vi "TapeDriveControllerCK_MasterSlave (3).vi"() -> ()   [LabVIEW 2011]
uses:
  <vilib>/Utility/error.llb/DialogType.ctl
  <instrlib>/Newport ESP301/Newport ESP301.lvlib
panel:
  out "level(ms)":dbl format="%.4g"
  in  "Tab Control":T1(tab)
  in  "Power Status":bool
  in  "Power Status 2":bool
  in  "Filename":string
  out "Slave Axis":i32
  out "Master Axis":i32
  in  "Release Slaving":bool
  in  "Switch Master Slave":bool
  in  "Interval":i32=1 min=1 max=1000
  in  "Reduction Ratio (0)":dbl min=-1000000.0 max=1000000.0 format="%.6g"
  in  "Turn OFF Slave":bool
  in  "Release Slaving\n after Discon":bool
  in  "VISA resource name":refnum<visa-resource-name>="COM1"
  in  "Connect":bool
  in  "Serial Link (RS232)":enum16{"RS232", "USB"}(ring)
  out "Connected?":bool
  in  "Save sinlge\nPicture":bool
  in  "Save all Shots":bool
  in  "Tab Control 2":T2(tab)=enum."Stepped Group"
  in  "Make Pictures":bool
  in  "Number of Steps":i32=5
  in  "Go steps":bool
  in  "Steplength(ms/mm)":dbl=10.0
  in  "Waittime":u32=800
  out "act. Step":u32=4
  in  "Wait befor picture(ms)":u32=50
  in  "Wait after picture(ms) 2":u32=100
  in  "Step Acc":dbl format="%.6f"
  in  "Step Velo":dbl min=-1000000.0 max=1000000.0 format="%.6g"
  in  "Go steps 2":bool
  in  "Waittime 2":u32
  in  "Wait after\n picture(ms) 2":u32
  out "act. Step 2":u32
  in  "Wait befor\n picture(ms) 2":u32
  in  "Steplength(ms) 2":u32
  in  "Number of Steps 2":i32
  in  "Make Pictures 2":bool
  in  "Stiff Velo":dbl min=-1000000.0 max=1000000.0 format="%.6g"
  in  "Stiff Acc":dbl format="%.6f"
  in  "Go steps 3":bool
  in  "1st Holdmove":dbl=20000.0
  in  "Steplength(ms) 3":dbl=10.0
  in  "Waittime 3":u32=1000
  in  "Wait befor\n picture(ms) 3":u32
  in  "Wait after\n picture(ms) 3":u32
  in  "Make Pictures 3":bool
  out "act. Step 3":u32
  in  "Number of Steps 3":i32=6
  in  "Motionphase":T3(array[cluster])=[{"Group Velocity (units/s)"=500.0, "Group Acceleration\n (0 units/s²) "=2000.0, "Group Vector Jerk\n (0 units/s^3)"=1000.0, "Group Decceleration \n(0 units/s²)"=4000.0, "Position (0 units)"=[50.0, 0.0], "groupInit Delay"=30}, {"Group Velocity (units/s)"=1000.0, "Group Acceleration\n (0 units/s²) "=2000.0, "Group Vector Jerk\n (0 units/s^3)"=4000.0, "Group Decceleration \n(0 units/s²)"=2000.0, "Position (0 units)"=[1000.0, 1000.0], "groupInit Delay"=10}]
  in  "StepMode":enum16{"Use Timing", "Use Encoder"}(ring)
  in  "E Stop":bool
  in  "AXIS":i32(ring)=1 items=["Axis1"=1, "Axis3"=3]
  out "Array":T4(array[cluster])
  in  "Acceleration (0 units/s²)":dbl min=0.0 format="%.4g"
  in  "Max Acceleration (0 units/s²)":dbl min=0.0 max=2000000000.0 format="%.6g"
  in  "Maximum Velocity (0 units/s)":dbl min=0.0 max=2000000000.0 format="%.6g"
  in  "Deceleration (0 units/s²)":dbl min=0.0 format="%.6g"
  in  "Velocity feed-forward gain factor (0)":dbl min=0.0 max=2000000000.0 format="%.6g"
  in  "Velocity (units/s)":dbl min=0.0 format="%.4g"
  in  "Acceleration feed-forward gain factor (0)":dbl min=0.0 max=2000000000.0 format="%.6g"
  in  "DAC Offset (0)":dbl min=-10.0 max=10.0 format="%.6g"
  out "DAC Offsets":dbl[](array[numeric]) format="%_6g"
  in  "Group Acceleration\n (0 units/s²)":dbl=4000.0 min=0.0 format="%.6g"
  in  "Group Velocity (units/s)":dbl=1000.0 min=0.0 format="%.4g"
  in  "Group Vector Jerk\n (0 units/s^3)":dbl=1000.0 min=0.0 max=2000000000.0 format="%.4g"
  in  "Group Decceleration \n(0 units/s²)":dbl=4000.0 min=0.0 format="%.6g"
  in  "Feedback Filter Settings":T5
  out "FilterSetup":T6(array[cluster])
  in  "Cluster":cluster{"Master Axis":i32, "Slave Axis":i32}={"Master Axis"=1, "Slave Axis"=3}
  in  "Encoder\nAxis":i32=2
  out "Remaining States":string
  in  "Get Relation of Slave":bool
  out "Slaves Master":i32
  out "Current State":string
  out "Reduction Ratio":dbl format="%.6g"
  out "Interval (ms)":i32
  in  "Motionphase 2":T3(array[cluster])
  in  "Group Move Comp":bool
  in  "Set Zero":bool
  out "Position (units)":dbl format="%.6g"
  in  "groupInit Delay":u32=50
  in  "Wait before read (0ms)":u32=100
  in  "Send Command":bool
  out "Answer":string
  in  "Command":string
  in  "End Program":bool
  in  "Group Mode":bool
  in  "MOVE MASTER":bool
  out "In Motion?":bool
  in  "MaxMotion":dbl=200000.0
  # "Debug Indicators"
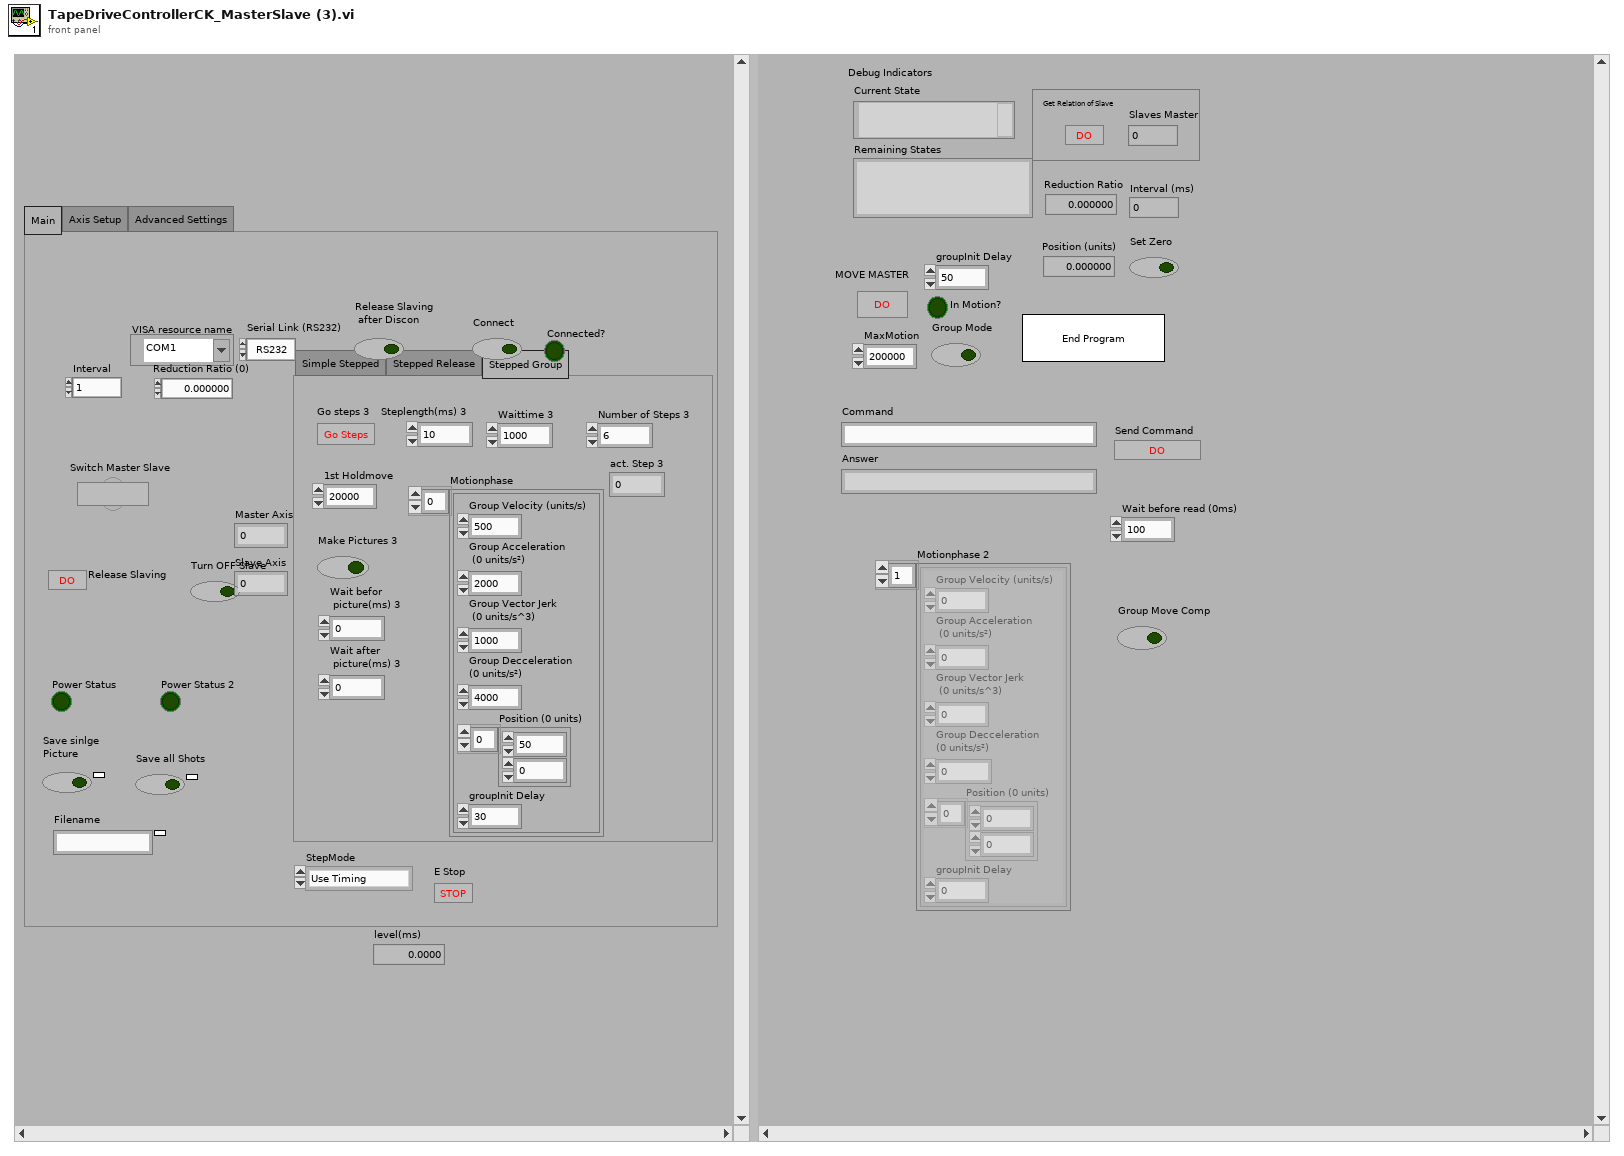
[diagram p1: front panel]
types:
  T1 = enum32{"Main", "Axis Setup", "Advanced Settings"}
  T2 = enum32{"Simple Stepped", "Stepped Release", "Stepped Group"}
  T3 = cluster{"Group Velocity (units/s)":dbl, "Group Acceleration\n (0 units/s²) ":dbl, "Group Vector Jerk\n (0 units/s^3)":dbl, "Group Decceleration \n(0 units/s²)":dbl, "Position (0 units)":dbl[], "groupInit Delay":u32}[]
  T4 = cluster{cluster{"Max Acceleration (units/s²)":dbl, "Maximum Velocity (units/s)":dbl, "Acceleration (units/s²)":dbl, "Deceleration (units/s²)":dbl, "Velocity (units/s)":dbl}, cluster{"Accel Gain":dbl, "Velocity Gain":dbl}}[]
  T5 = cluster{"Ks (0)":dbl, "Ki (0)":dbl, "Kp (0)":dbl, "Kd (0)":dbl}
  T6 = cluster{"Ks":dbl, "Kp":dbl, "Ki":dbl, "Kd":dbl}[]
  T7 = enum32{"invalid app kind", "Development System", "Run Time System", "Student Edition", "Embedded LabVIEW", "Evaluation", "Custom"}
  T8 = enum32{"Invalid", "Standard", "Closed", "Hidden", "Minimized", "Maximized"}
  T9 = enum16{"Trapezoidal Mode", "S-curve Mode", "Jog Mode", "Slave to master's desired position (trajectory)", "Slave to master's actual position (feedback)", "Slave to master's actual velocity for jogging"}
  T10 = cluster{"Grouped?":bool, "Master Axis":i32, "Group Number (1)":i32}
  T11 = cluster{"Core":cluster{"Current VI Reference":refnum<vi>, "Close Panel on Exit?":bool}, "VISA resource name":refnum<visa-resource-name>, "Velocity (units/s)":dbl, "Acceleration (0 units/s²)":dbl, "Connected?":bool, "Master Axis":i32, "Slave Axis":i32, "In Motion?":bool, "Stepper Cluster":cluster{"Stepped Motion":bool, "Moving":bool, "millisecond timer value":u32, "act. Step":u32}, "Stepper Cluster 2":cluster{"Stepped Motion":bool, "Moving":bool, "millisecond timer value":u32, "act. Step":u32}, "Group Cluster":cluster{"Grouped?":bool, "Master Axis":i32, "Group Number (1)":i32}, "Stepper Cluster 3":cluster{"Stepped Motion":bool, "Moving":bool, "millisecond timer value":u32, "act. Step":u32}, "Stepper Cluster 4":cluster{"Stepped Motion":bool, "Moving":bool, "millisecond timer value":u32, "act. Step":u32}, "actual Position":dbl, "Last Position":dbl}
  T12 = typedef "DialogType.ctl" = u16
  T13 = cluster{"Stepped Motion":bool, "Moving":bool, "millisecond timer value":u32, "act. Step":u32}
  T14 = cluster{"Current VI Reference":refnum<vi>, "Close Panel on Exit?":bool}
  T15 = cluster{"Acceleration (units/s²)":dbl, "Maximum Velocity (units/s)":dbl, "Acceleration (units/s²)":dbl, "Deceleration (units/s²)":dbl, "Velocity (units/s)":dbl}
  T16 = cluster{cluster{"Acceleration (units/s²)":dbl, "Maximum Velocity (units/s)":dbl, "Acceleration (units/s²)":dbl, "Deceleration (units/s²)":dbl, "Velocity (units/s)":dbl}, cluster{"Gain":dbl, "Gain":dbl}}
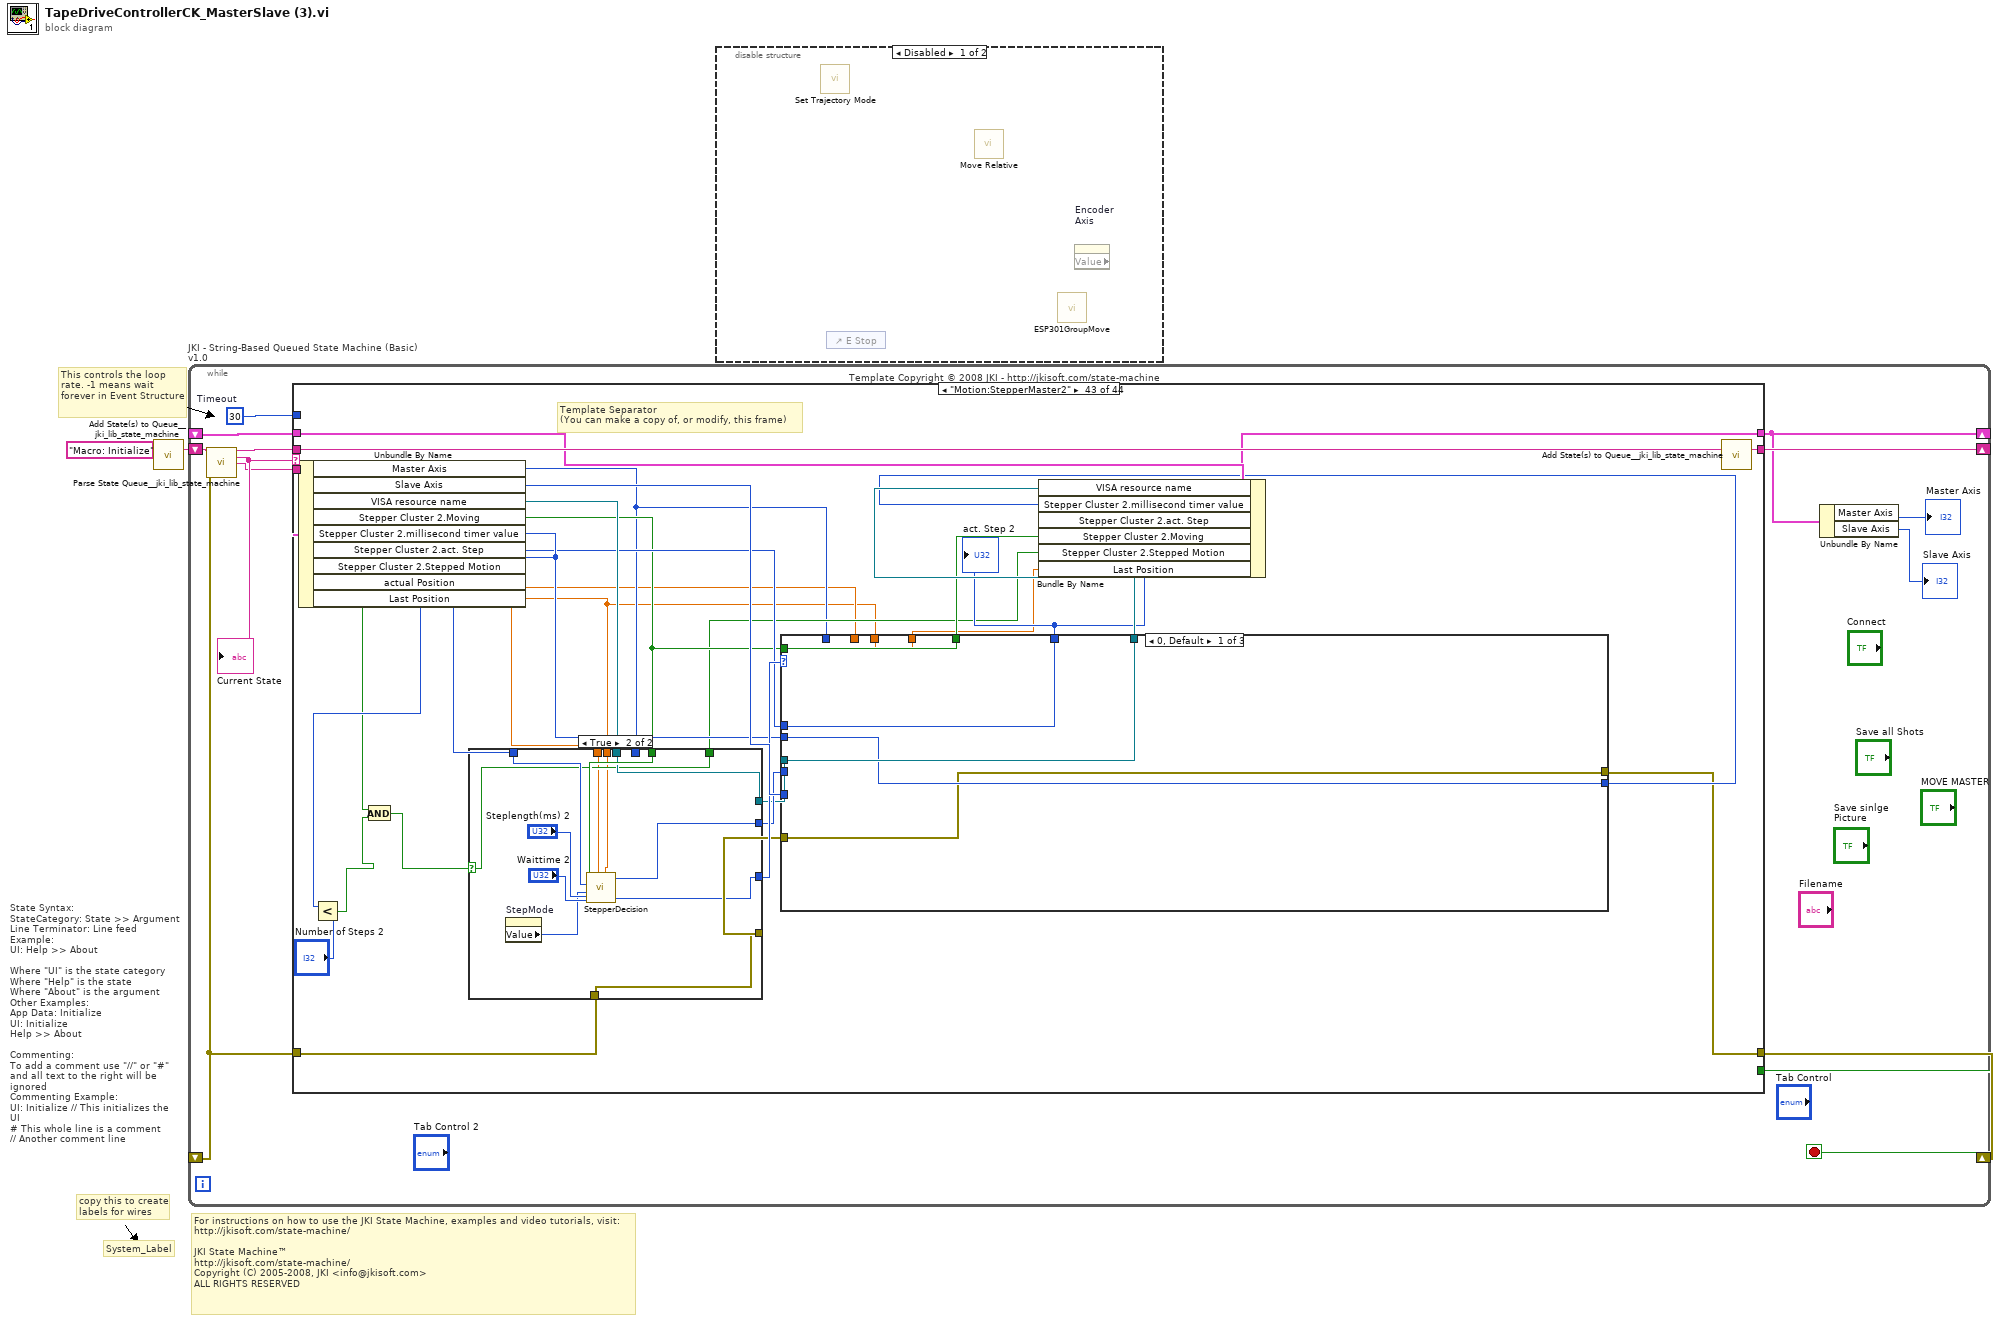
[diagram p0: block diagram]
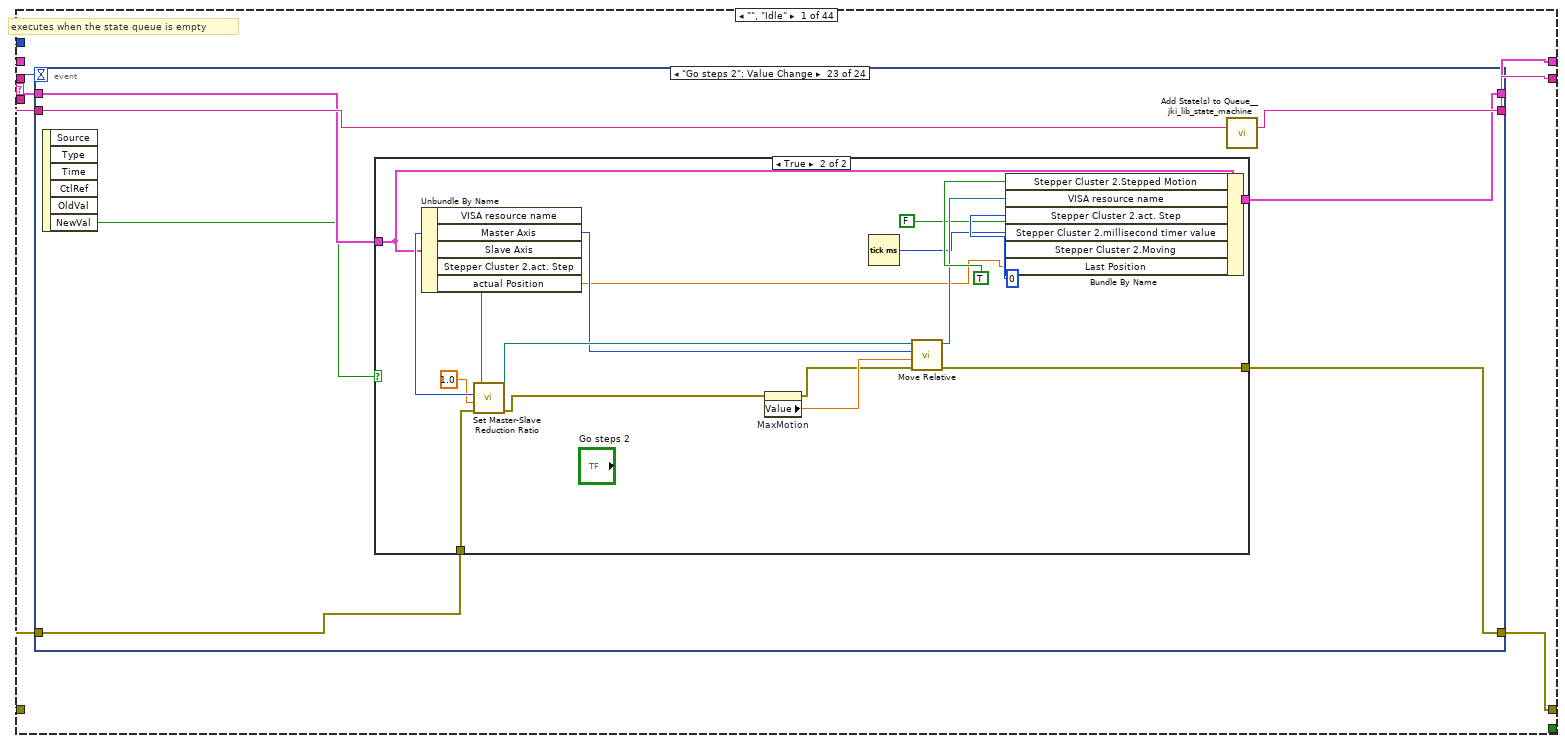
[diagram p3: hidden frame]
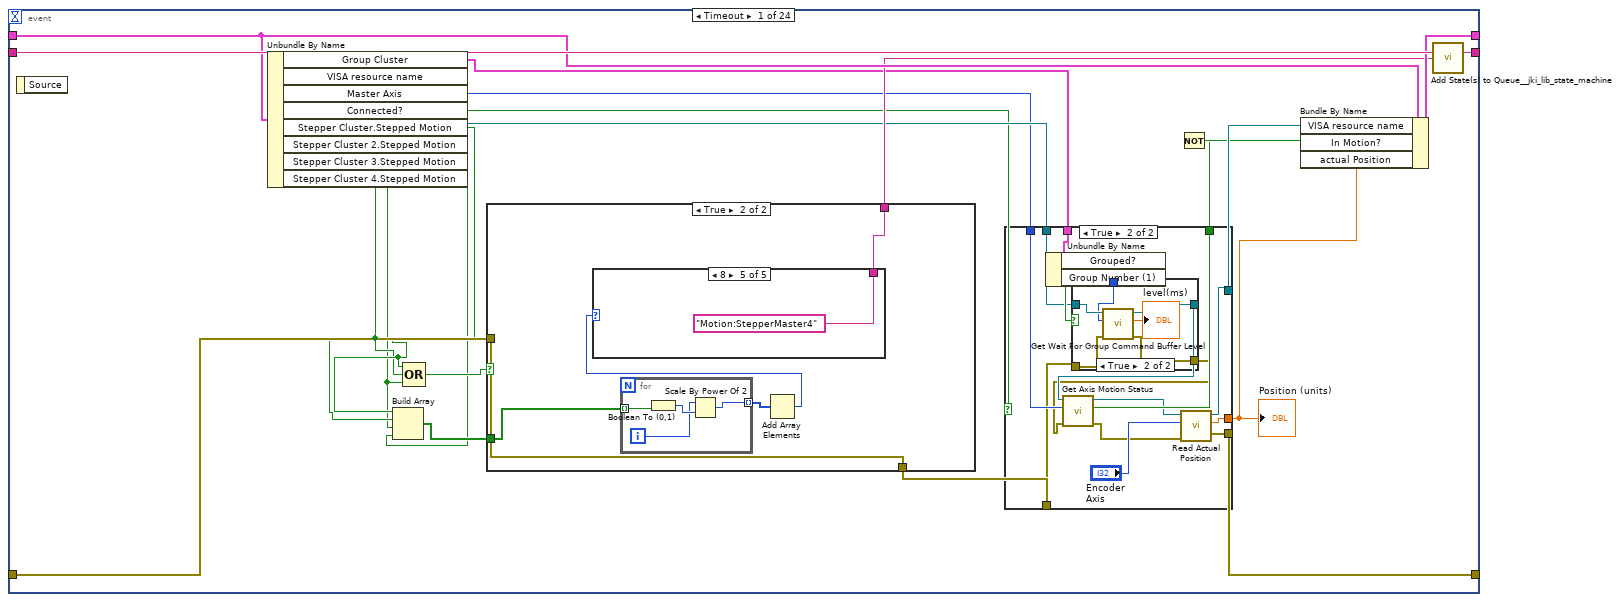
[diagram p4: hidden frame]
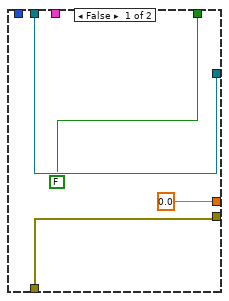
[diagram p5: hidden frame]
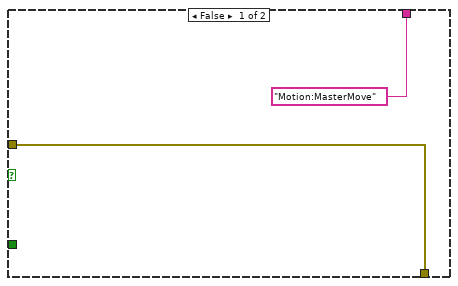
[diagram p7: hidden frame]
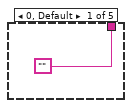
[diagram p8: hidden frame]
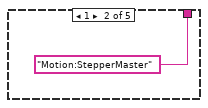
[diagram p9: hidden frame]
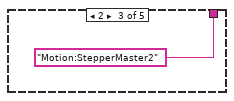
[diagram p10: hidden frame]
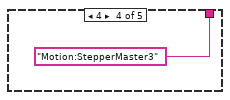
[diagram p11: hidden frame]
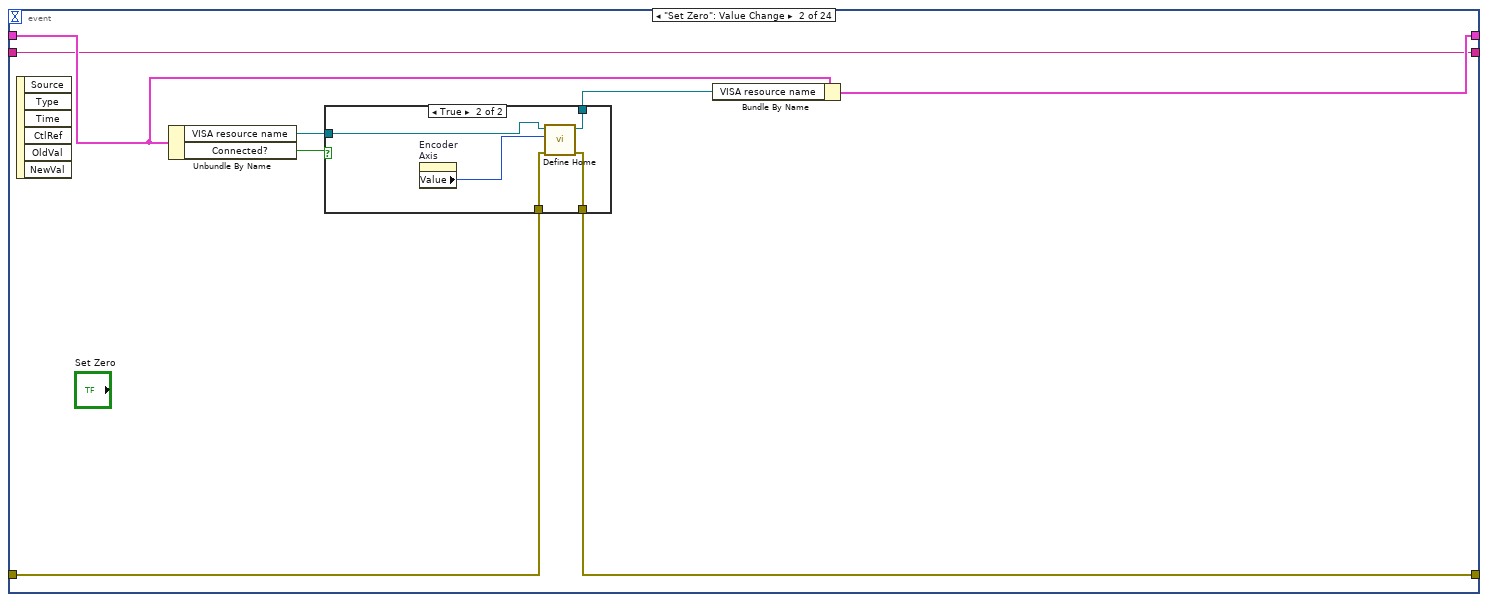
[diagram p12: hidden frame]
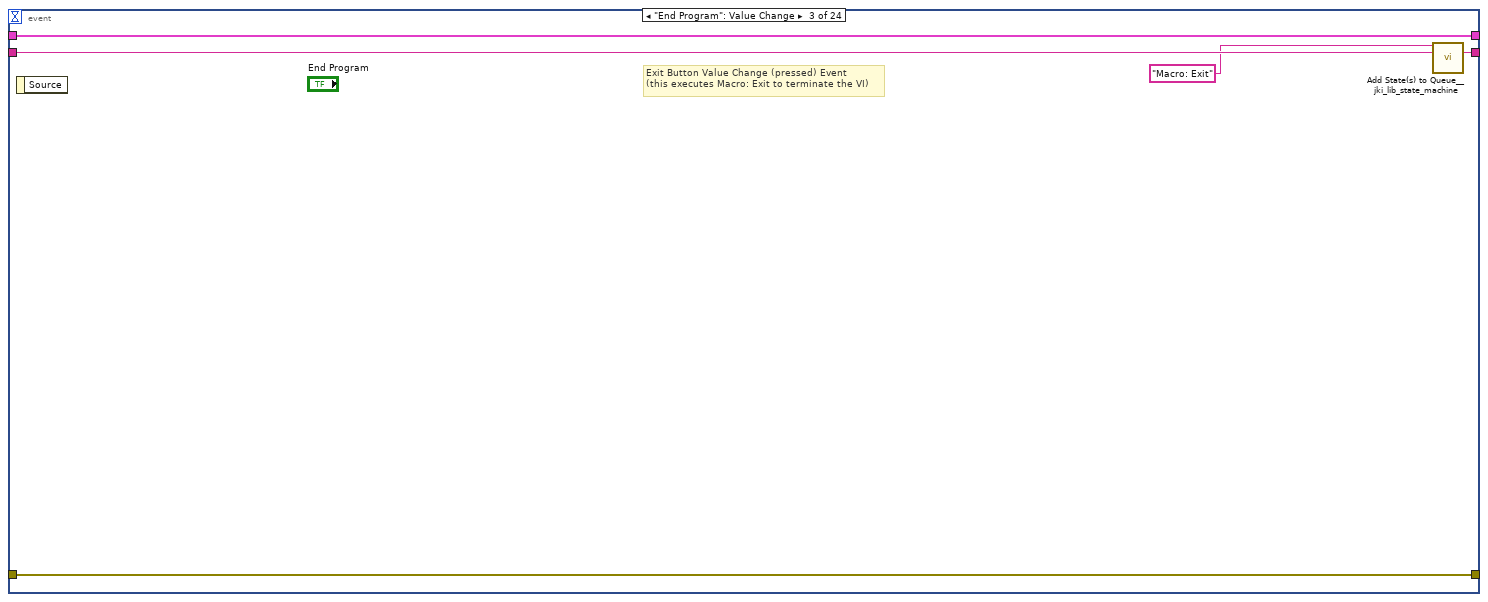
[diagram p14: hidden frame]
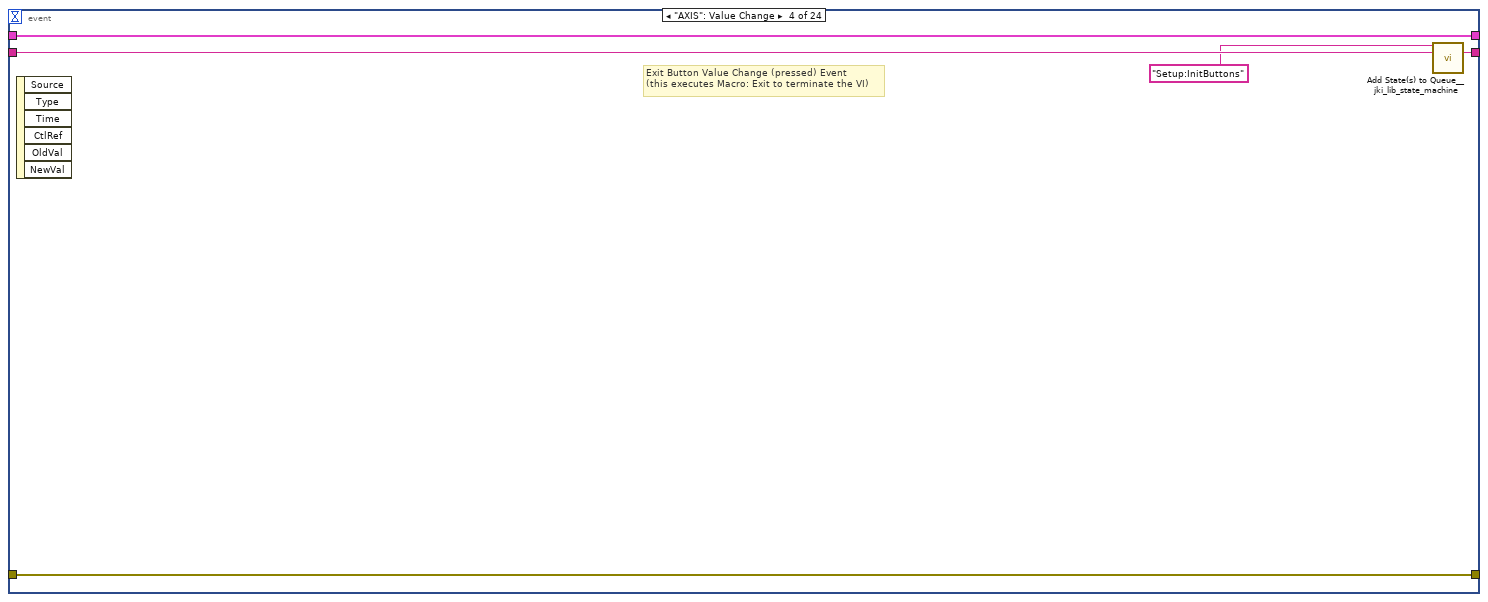
[diagram p15: hidden frame]
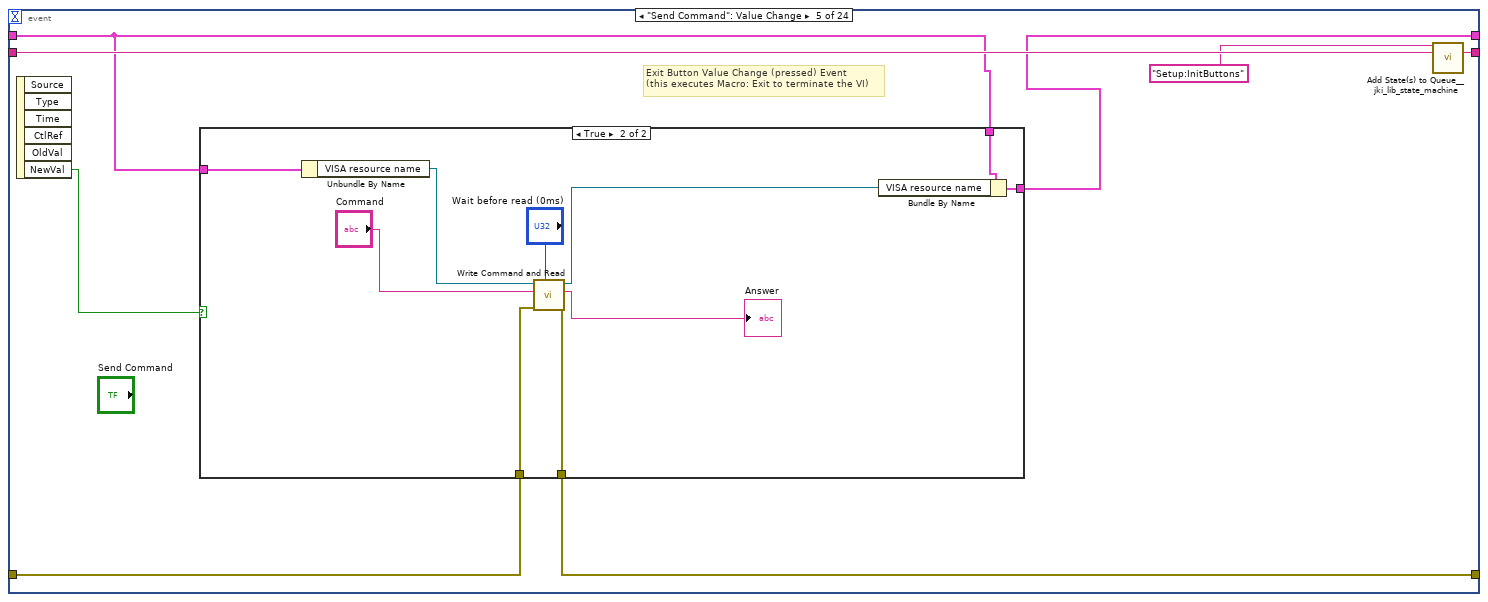
[diagram p16: hidden frame]
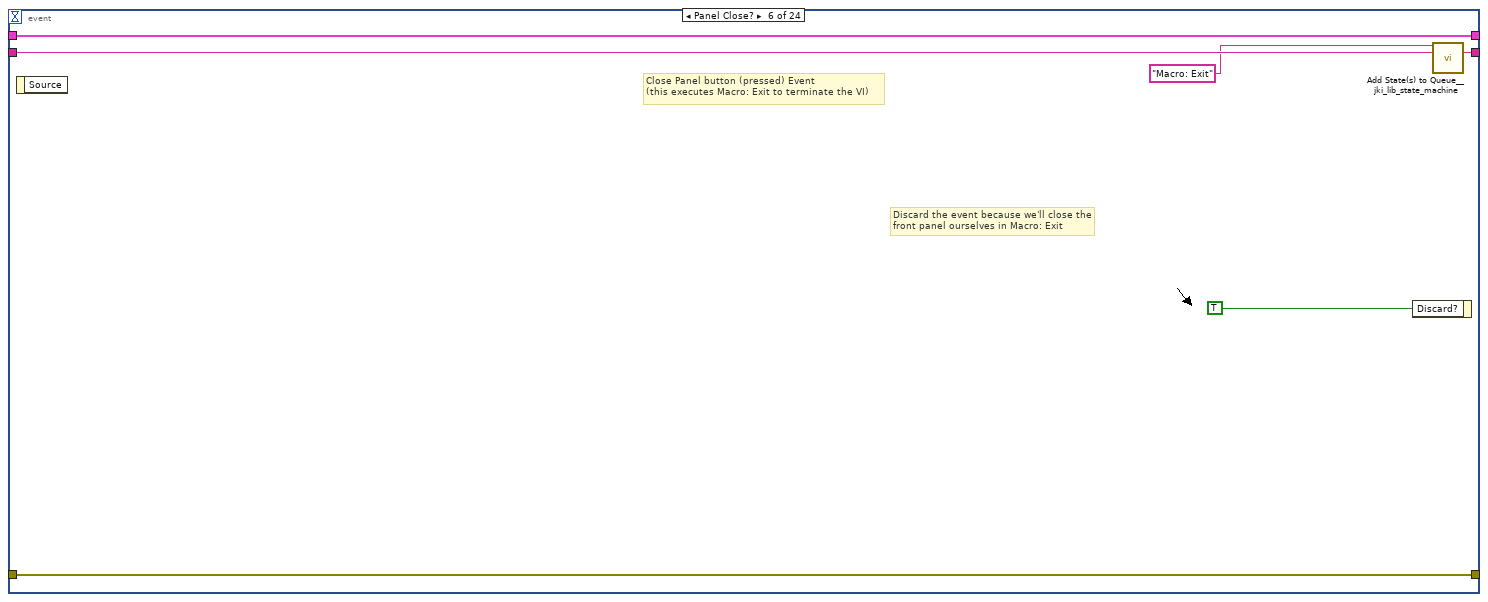
[diagram p18: hidden frame]
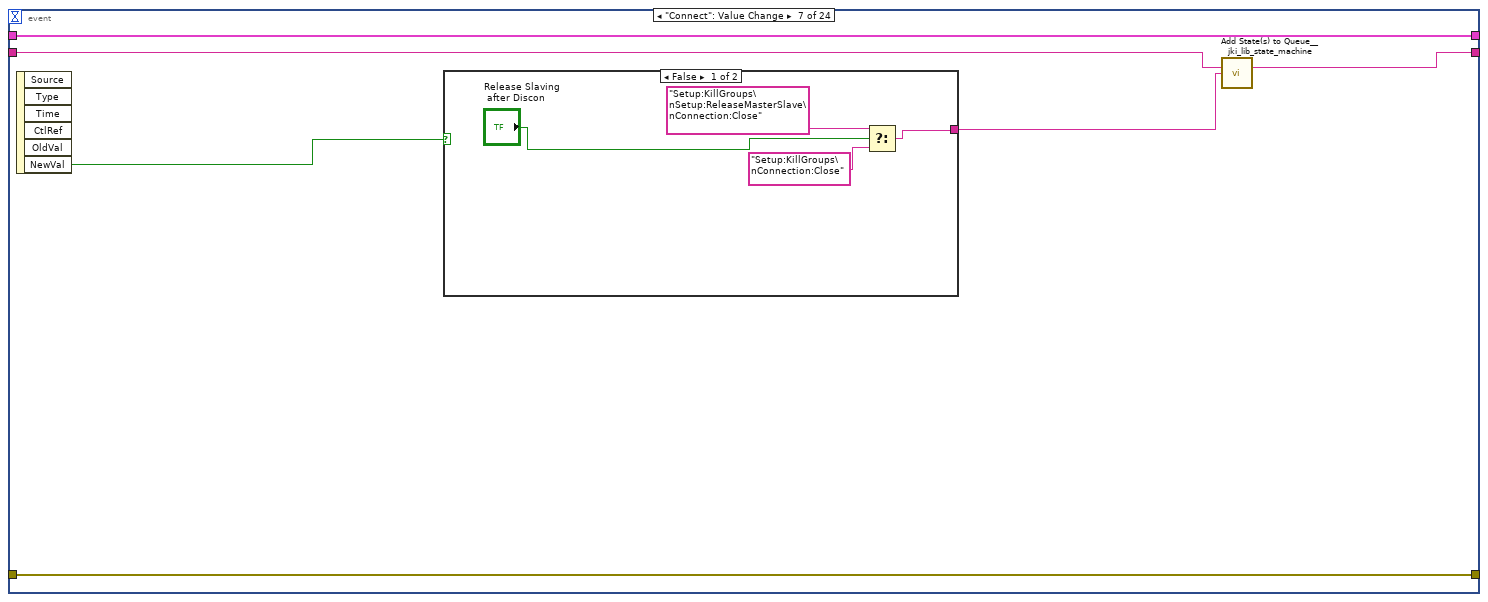
[diagram p19: hidden frame]
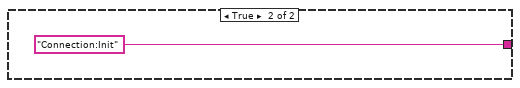
[diagram p20: hidden frame]
diagram:
  # "For instructions on how to use the JKI State Machine, examples and video tutorials, visit:\nhttp://jkisoft.com/state-machine/\n\nJKI State Machine™\nhttp://jkisoft.com/state-machine/\nCopyright (C) 2005-2008, JKI <info@jkisoft.com>\nALL RIGHTS RESERVED"
  # "State Syntax:\nStateCategory: State >> Argument\nLine Terminator: Line feed\nExample:\nUI: Help >> About\n\nWhere \"UI\" is the state category\nWhere \"Help\" is the state\nWhere \"About\" is the argument\nOther Examples:\nApp Data: Initialize\nUI: Initialize\nHelp >> About\n\nCommenting:\nTo add a comment use \"//\" or \"#\" and all text to the right will be ignored\nCommenting Example:\nUI: Initialize // This initializes the UI\n# This whole line is a comment\n// Another comment line"
  # "copy this to create labels for wires"
  # "This controls the loop rate. -1 means wait forever in Event Structure"
  # "System_Label"
  n1 = call <vilib>:"Add State(s) to Queue__jki_lib_state_machine.vi"("State(s) in (\"\")"="Macro: Initialize") -> ("States Out"=w2:string)  [unwired: 14 in]
  n2 = while "JKI - String-Based Queued State Machine (Basic) v1.0" {
    shift-right: [w5] -> _
    shift-left: _ -> [w8]
    shift-right: [w11] -> _
    shift-left: _ -> [w6]
    shift-right: [w10] -> _
    shift-left: w2 -> [w12]
    stop <- w9 stop-if-true
    w7 = 30  # Timeout
    # "Template Copyright © 2008 JKI - http://jkisoft.com/state-machine"
    n3 = call <vilib>:"Parse State Queue__jki_lib_state_machine.vi"("State Queue"=w12, "Error In (no error)"=w6) -> ("Remaining States"=w14:string, "Current State"=w15:string, "Arguments"=w13:string)  [unwired: 11 in]
    "Current State" <- w15
    n4 = case shown="\"Motion:StepperMaster2\"" w15 {
      selector: w15 -> [_ _ w419 _ _ _ _ _ _ _ _ _ _ _ _ _ _ _ _ _ _ _ _ _ _ _ _ _ _ _ _ _ _ _ _ _ _ _ _ _ _ _ _ _]
      tunnel: w14 -> [w22 w418 w423 w441 w448 w453 w457 w477 w483 w487 w508 w514 w525 w551 w556 w573 w577 w591 w603 w621 w633 w649 w662 w683 w717 w731 w772 w819 w828 w851 w882 w965 w999 w1037 w1050 w1071 w1073 w1095 w1113 w1117 w1131 w1187 w1284 w1391]
      tunnel: w13 -> [_ _ _ _ _ _ _ _ _ _ _ w509 w519 _ _ _ _ w583 _ _ w630 _ w654 _ _ _ _ _ _ _ _ _ _ _ _ _ _ _ _ _ _ _ _ _]
      tunnel: w8 -> [w20 w415 w421 w432 w445 w451 w454 _ w479 w484 w494 w512 w521 w548 w553 w570 w574 w587 w601 w619 w631 w645 w660 w681 w715 w729 w770 w817 w826 w849 w880 w963 w997 w1032 w1048 w1068 w1076 w1090 w1111 w1114 w1128 w1185 w1282 w1389]
      tunnel: [w19 w416 w425 w438 errorcluster {"status"=FALSE, "code"=0, "source"=""} ("error out") w450 w455 w474 w480 w485 w495 w510 w522 w549 w554 w571 w575 w579 w597 w609 w628 w634 w656 w676 w703 w725 w766 w789 w821 w844 w873 w958 w992 w1016 w1038 w1069 w1072 w1091 w1109 w1115 w1122 w1177 w1274 w1381] -> w11
      tunnel: w6 -> [w18 w416 w424 w438 w444 w450 w455 w474 w478 w485 w496 w511 w523 w549 w554 w571 w575 w580 w596 w617 w628 w641 w657 w679 w711 w727 w768 w815 w823 w846 w876 w960 w994 w1030 w1044 w1069 w1077 w1093 w1106 w1115 w1123 w1172 w1270 w1377]
      tunnel: [w21 w417 w422 w440 w447 w452 w456 w476 w482 w486 w507 w513 w524 w550 w555 w572 w576 w590 w602 w620 w632 w648 w661 w682 w716 w730 w771 w818 w827 w850 w881 w964 w998 w1036 w1049 w1070 w1079 w1094 w1112 w1116 w1130 w1186 w1283 w1390] -> w10
      tunnel: [_ _ _ _ _ TRUE _ _ _ _ _ _ _ _ _ _ _ _ _ _ _ _ _ _ _ _ _ _ _ _ _ _ _ _ _ _ _ _ _ _ _ _ _ _] -> w9
      tunnel: [w17 w415 w421 w439 w445 w451 w454 w475 w479 w484 w493 w512 w521 w548 w553 w570 w574 w586 w600 w618 w631 w644 w659 w680 w714 w728 w769 w816 w825 w848 w879 w962 w996 w1031 w1047 w1068 w1075 w1089 w1110 w1114 w1129 w1184 w1281 w1388] -> w5
      tunnel: w7 -> [w16 _ _ _ _ _ _ _ _ _ _ _ _ _ _ _ _ _ _ _ _ _ _ _ _ _ _ _ _ _ _ _ _ _ _ _ _ _ _ _ _ _ _ _]
      frame "", "Idle" {
        # "executes when the state queue is empty"
        n5 = event shown="[22] \"Go steps 2\": Value Change" {
          selector: _ -> [_ _ _ _ _ _ _ _ _ _ _ _ _ _ _ _ _ _ _ _ _ _ _ _]
          dyn-events: _ -> [_ _ _ _ _ _ _ _ _ _ _ _ _ _ _ _ _ _ _ _ _ _ _ _]
          timeout: w16 -> [_ _ _ _ _ _ _ _ _ _ _ _ _ _ _ _ _ _ _ _ _ _ _ _]
          tunnel: w22 -> [w44 w93 w107 w112 w120 w138 w142 w153 w158 w171 w176 w183 w193 w214 w219 w226 w235 w269 w286 w302 w318 w325 w354 w383]
          tunnel: [w43 w93 w106 w111 w119 w137 w140 w151 w157 w170 w174 w181 w192 w214 w218 w225 w236 w270 w287 w303 w319 w326 w355 w384] -> w21
          tunnel: w20 -> [w42 w95 w104 w109 w115 w135 w143 w154 w159 w165 w177 w184 w190 w208 w221 w228 w232 w267 w283 w300 w316 w324 w353 w382]
          tunnel: [w32 w91 w105 w110 w113 w136 w139 w150 w156 w160 w173 w180 w191 w210 w216 w223 w230 w263 w275 w288 w304 w321 w350 w379] -> w19
          tunnel: w18 -> [w40 w92 w105 w110 w114 w136 w139 w150 w156 w161 w173 w180 w191 w211 w216 w223 w231 w263 w276 w289 w305 w322 w351 w380]
          tunnel: [w41 w94 w104 w109 w116 w135 w143 w154 w159 w164 w177 w184 w189 w207 w220 w227 w234 w268 w285 w299 w315 w323 w352 w381] -> w17
          event Timeout {
            n6 = event-data() -> ()  [unwired: 1 in, 1 out]
            n7 = Unbundle By Name(w42) -> ("Group Cluster"=w23:T10, "VISA resource name"=w31:refnum<visa-resource-name>, "Master Axis"=w28:i32, "Connected?"=w25:bool, "Stepper Cluster.Stepped Motion"=w37:bool, "Stepper Cluster 2.Stepped Motion"=w36:bool, "Stepper Cluster 3.Stepped Motion"=w35:bool, "Stepper Cluster 4.Stepped Motion"=w29:bool)
            n8 = Build Array(w37, w36, w35, w29) -> (w34:bool[])
            n9 = Compound Arithmetic op=OR(w37, w36, w35) -> (w38:bool)
            n10 = case shown="True" w38 {
              tunnel: w40 -> [w72 w78]
              tunnel: [w72 w78] -> w33
              tunnel: ["Motion:MasterMove" w74] -> w39
              tunnel: w34 -> [_ w77]
              frame False {
              }
              frame True {
                n11 = for {
                  tunnel: w77 -> [w87] mode=indexing
                  tunnel: [w84] -> w76 mode=indexing
                  i -> [w85]
                  n12 = Boolean To (0,1)(Boolean=w87) -> (0, 1=w86:i16)
                  n13 = Scale By Power Of 2(n=w85, x=w86) -> (x*2^n=w84:i16)
                }
                n14 = Add Array Elements(numeric array=w76) -> (sum=w75:i16)
                n15 = case shown="8" w75 {
                  tunnel: ["" "Motion:StepperMaster" ("State(s) at Back (\"\")") "Motion:StepperMaster2" ("State(s) at Back (\"\")") "Motion:StepperMaster3" ("State(s) at Back (\"\")") "Motion:StepperMaster4" ("State(s) at Back (\"\")")] -> w74
                  frame 0, Default {
                  }
                  frame 1 {
                  }
                  frame 2 {
                  }
                  frame 4 {
                  }
                  frame 8 {
                  }
                }
              }
            }
            n16 = case shown="True" w25 {
              tunnel: w33 -> [w47 w51]
              tunnel: [w47 w60] -> w32
              tunnel: w31 -> [w48 w53]
              tunnel: [w48 w56] -> w30
              tunnel: [0.0 ("Position (units)") w62] -> w24
              tunnel: w28 -> [_ w59]
              tunnel: [FALSE ("Motion Done") w58] -> w26
              tunnel: w23 -> [_ w55]
              frame False {
              }
              frame True {
                n17 = Unbundle By Name(w55) -> ("Grouped?"=w54:bool, "Group Number (1)"=w49:i32)
                n18 = case shown="True" w54 {
                  tunnel: w53 -> [w65 w71]
                  tunnel: [w65 w70] -> w52
                  tunnel: w51 -> [w64 w68]
                  tunnel: [w64 w67] -> w50
                  tunnel: w49 -> [_ w66]
                  frame False {
                  }
                  frame True {
                    n19 = call <instrlib>:"Get Wait For Group Command Buffer Level.vi"("error in (no error)"=w68, "Group Number (1)"=w66, "VISA resource name"=w71) -> ("error out"=w67:errorcluster, "level(ms)"=→"level(ms)":dbl, "VISA resource name out"=w70:refnum<visa-resource-name>)  [unwired: 2 in]
                  }
                }
                n20 = call <instrlib>:"Get Axis Motion Status.vi"("error in (no error)"=w50, "Axis (1)"=w59, "VISA resource name"=w52) -> ("error out"=w61:errorcluster, "Motion Done"=w58:bool, "VISA resource name out"=w57:refnum<visa-resource-name>)  [unwired: 2 in]
                n21 = call <instrlib>:"Read Actual Position.vi"("error in (no error)"=w61, "Axis (1)"="Encoder\nAxis", "VISA resource name"=w57) -> ("error out"=w60:errorcluster, "Position (units)"=w62:dbl, "VISA resource name out"=w56:refnum<visa-resource-name>)  [unwired: 2 in]
              }
            }
            "Position (units)" <- w24
            n22 = Not(x=w26) -> (.not. x?=w27:bool)
            n23 = Bundle By Name(cluster=w42, "VISA resource name"=w30, "In Motion?"=w27, "actual Position"=w24) -> (w41:T11)
            n24 = call <vilib>:"Add State(s) to Queue__jki_lib_state_machine.vi"("State(s) in (\"\")"=w44, "State(s) at Back (\"\")"=w39) -> ("States Out"=w43:string)  [unwired: 13 in]
          }
          event "Set Zero": Value Change {
            n25 = event-data() -> ()  [unwired: 1 in, 6 out]
            n26 = Unbundle By Name(w95) -> ("VISA resource name"=w90:refnum<visa-resource-name>, "Connected?"=w88:bool)
            n27 = case shown="True" w88 {
              tunnel: w92 -> [w96 w102]
              tunnel: [w96 w101] -> w91
              tunnel: w90 -> [w97 w100]
              tunnel: [w97 w99] -> w89
              frame False {
              }
              frame True {
                n28 = property on="Encoder\nAxis" class="DigNum (strict)"() -> ("Value"=w98:i32)  [unwired: 2 in, 2 out]
                n29 = call <instrlib>:"Define Home.vi"("error in (no error)"=w102, "Axis (1)"=w98, "VISA resource name"=w100) -> ("error out"=w101:errorcluster, "VISA resource name out"=w99:refnum<visa-resource-name>)  [unwired: 3 in]
              }
            }
            n30 = Bundle By Name(cluster=w95, "VISA resource name"=w89) -> (w94:T11)
          }
          event "End Program": Value Change {
            # "Exit Button Value Change (pressed) Event\n(this executes Macro: Exit to terminate the VI)"
            n31 = event-data() -> ()  [unwired: 1 in, 1 out]
            n32 = call <vilib>:"Add State(s) to Queue__jki_lib_state_machine.vi"("State(s) in Front (\"\")"="Macro: Exit", "State(s) in (\"\")"=w107) -> ("States Out"=w106:string)  [unwired: 13 in]
          }
          event "AXIS": Value Change {
            # "Exit Button Value Change (pressed) Event\n(this executes Macro: Exit to terminate the VI)"
            n33 = event-data() -> ()  [unwired: 1 in, 6 out]
            n34 = call <vilib>:"Add State(s) to Queue__jki_lib_state_machine.vi"("State(s) in Front (\"\")"="Setup:InitButtons", "State(s) in (\"\")"=w112) -> ("States Out"=w111:string)  [unwired: 13 in]
          }
          event "Send Command": Value Change {
            # "Exit Button Value Change (pressed) Event\n(this executes Macro: Exit to terminate the VI)"
            n35 = event-data() -> ("NewVal"=w117:bool)  [unwired: 1 in, 5 out]
            n36 = case shown="True" w117 {
              tunnel: w115 -> [w122 w131]
              tunnel: [w122 w130] -> w116
              tunnel: w115 -> [_ w129]
              tunnel: w114 -> [w121 w124]
              tunnel: [w121 w123] -> w113
              frame False {
              }
              frame True {
                n37 = Unbundle By Name(w129) -> ("VISA resource name"=w128:refnum<visa-resource-name>)
                n38 = call <instrlib>:"Write Command and Read.vi"("Wait before read (0ms)"="Wait before read (0ms)", "error in (no error)"=w124, "Command"="Command", "VISA resource name"=w128) -> ("error out"=w123:errorcluster, "Returned string"=→"Answer":string, "VISA resource name out"=w127:refnum<visa-resource-name>)  [unwired: 3 in]
                n39 = Bundle By Name(cluster=w131, "VISA resource name"=w127) -> (w130:T11)
              }
            }
            n40 = call <vilib>:"Add State(s) to Queue__jki_lib_state_machine.vi"("State(s) in Front (\"\")"="Setup:InitButtons", "State(s) in (\"\")"=w120) -> ("States Out"=w119:string)  [unwired: 13 in]
          }
          event Panel Close? {
            # "Discard the event because we'll close the front panel ourselves in Macro: Exit"
            # "Close Panel button (pressed) Event\n(this executes Macro: Exit to terminate the VI)"
            n41 = event-data() -> ()  [unwired: 1 in, 1 out]
            n42 = event-data("Discard?"=TRUE) -> ()  [unwired: 1 in, 1 out]
            n43 = call <vilib>:"Add State(s) to Queue__jki_lib_state_machine.vi"("State(s) in Front (\"\")"="Macro: Exit", "State(s) in (\"\")"=w138) -> ("States Out"=w137:string)  [unwired: 13 in]
          }
          event "Connect": Value Change {
            n44 = event-data() -> ("NewVal"=w144:bool)  [unwired: 1 in, 5 out]
            n45 = case shown="False" w144 {
              tunnel: [w145 "Connection:Init"] -> w141
              frame False {
                n46 = Select(t="Setup:KillGroups\nSetup:ReleaseMasterSlave\nConnection:Close", s="Release Slaving\n after Discon", f="Setup:KillGroups\nConnection:Close") -> (s? t:f=w145:string)
              }
              frame True {
              }
            }
            n47 = call <vilib>:"Add State(s) to Queue__jki_lib_state_machine.vi"("State(s) in (\"\")"=w142, "State(s) at Back (\"\")"=w141) -> ("States Out"=w140:string)  [unwired: 13 in]
          }
          event "Cluster": Value Change {
            n48 = event-data() -> ()  [unwired: 1 in, 6 out]
            n49 = call <vilib>:"Add State(s) to Queue__jki_lib_state_machine.vi"("State(s) in (\"\")"=w153, "State(s) at Back (\"\")"="Connection:Init") -> ("States Out"=w151:string)  [unwired: 13 in]
          }
          event "DAC Offset (0)": Value Change {
            n50 = event-data() -> ()  [unwired: 1 in, 6 out]
            n51 = call <vilib>:"Add State(s) to Queue__jki_lib_state_machine.vi"("State(s) in (\"\")"=w158, "State(s) at Back (\"\")"="Setup:MotorONOFF>>OFF\nSetup:Wait>>1000\nSetup:SetDACOffset\nSetup:MotorONOFF>>ON") -> ("States Out"=w157:string)  [unwired: 13 in]
          }
          event "Feedback Filter Settings": Value Change {
            n52 = event-data() -> ()  [unwired: 1 in, 6 out]
            n53 = Unbundle By Name(w165) -> ("VISA resource name"=w166:refnum<visa-resource-name>)
            n54 = property on="AXIS" class="Ring (strict)"() -> ("Value"=w162:i32)  [unwired: 2 in, 2 out]
            n55 = call "Update_FBFilter.vi"("Axis"=w162, "error in (no error)"=w161, "Disable?"=enum16{"Disable", "Set"}."Set", "Feedback Filter Settings"="Feedback Filter Settings", "VISA resource name"=w166) -> ("error out"=w160:errorcluster, "VISA resource name out"=w163:refnum<visa-resource-name>)  [unwired: 5 in]
            n56 = Bundle By Name(cluster=w165, "VISA resource name"=w163) -> (w164:T11)
            n57 = call <vilib>:"Add State(s) to Queue__jki_lib_state_machine.vi"("State(s) in (\"\")"=w171, "State(s) at Back (\"\")"="Setup:RBFBFilter") -> ("States Out"=w170:string)  [unwired: 13 in]
          }
          event "Release Slaving": Value Change {
            n58 = event-data() -> ("NewVal"=w172:bool)  [unwired: 1 in, 5 out]
            n59 = case shown="True" w172 {
              tunnel: ["" "Setup:ReleaseMasterSlave"] -> w175
              frame False {
              }
              frame True {
              }
            }
            n60 = call <vilib>:"Add State(s) to Queue__jki_lib_state_machine.vi"("State(s) in (\"\")"=w176, "State(s) at Back (\"\")"=w175) -> ("States Out"=w174:string)  [unwired: 13 in]
          }
          event "Interval", "Reduction Ratio (0)": Value Change {
            n61 = event-data() -> ()  [unwired: 1 in, 6 out]
            n62 = call <vilib>:"Add State(s) to Queue__jki_lib_state_machine.vi"("State(s) in (\"\")"=w183, "State(s) at Back (\"\")"="Setup:Speed") -> ("States Out"=w181:string)  [unwired: 13 in]
          }
          event "Switch Master Slave": Value Change {
            n63 = event-data() -> ()  [unwired: 1 in, 6 out]
            n64 = Unbundle By Name(w190) -> ("Master Axis"=w188:i32, "Slave Axis"=w187:i32, "Group Cluster.Grouped?"=w185:bool)
            n65 = case shown="False" w185 {
              tunnel: [w197 ""] -> w186
              frame False {
                n66 = Concatenate Strings("\r\n", "Setup:SlaveOFF" ("string")) -> (w201:string)
                n67 = Select(t=w201, s="Turn OFF Slave", f="") -> (s? t:f=w198:string)
                n68 = Concatenate Strings("\r\n", "Setup:RBMotorPower" ("string")) -> (w194:string)
                n69 = Concatenate Strings("Setup:MotorONOFF>>OFF\nSetup:ReleaseMasterSlave\nSetup:Wait>>50\nSetup:MasterSlave\nSetup:Speed\nSetup:MotorONOFF>>ON", w198, w194) -> (w197:string)
              }
              frame True {
              }
            }
            n70 = Bundle By Name(cluster=w190, "Master Axis"=w187, "Slave Axis"=w188) -> (w189:T11)
            n71 = call <vilib>:"Add State(s) to Queue__jki_lib_state_machine.vi"("State(s) in (\"\")"=w193, "State(s) at Back (\"\")"=w186) -> ("States Out"=w192:string)  [unwired: 13 in]
          }
          event "Get Relation of Slave": Value Change {
            n72 = event-data() -> ()  [unwired: 1 in, 6 out]
            n73 = Unbundle By Name(w208) -> ("VISA resource name"=w213:refnum<visa-resource-name>, "Slave Axis"=w212:i32)
            n74 = call <instrlib>:"Get Master-Slave Relationship.vi"("error in (no error)"=w211, "Slave Axis"=w212, "VISA resource name"=w213) -> ("error out"=w210:errorcluster, "Master Axis"=→"Slaves Master":i32, "VISA resource name out"=w206:refnum<visa-resource-name>)  [unwired: 2 in]
            n75 = Bundle By Name(cluster=w208, "VISA resource name"=w206) -> (w207:T11)
          }
          event "Acceleration feed-forward gain factor (0)", "Velocity feed-forward gain factor (0)": Value Change {
            n76 = event-data() -> ()  [unwired: 1 in, 6 out]
            n77 = Unbundle By Name(w221) -> ("VISA resource name"=w215:refnum<visa-resource-name>)
            n78 = Bundle By Name(cluster=w221, "VISA resource name"=w215) -> (w220:T11)
            n79 = call <vilib>:"Add State(s) to Queue__jki_lib_state_machine.vi"("State(s) in (\"\")"=w219, "State(s) at Back (\"\")"="Setup:PIDFilter\nSetup:RBSetup" ("State(s) at Back (\"\")")) -> ("States Out"=w218:string)  [unwired: 13 in]
          }
          event "Maximum Velocity (0 units/s)", "Max Acceleration (0 units/s²)", "Acceleration (0 units/s²)", "Deceleration (0 units/s²)", "Velocity (units/s)": Value Change {
            n80 = event-data() -> ()  [unwired: 1 in, 6 out]
            n81 = Unbundle By Name(w228) -> ("VISA resource name"=w222:refnum<visa-resource-name>)
            n82 = Bundle By Name(cluster=w228, "VISA resource name"=w222) -> (w227:T11)
            n83 = call <vilib>:"Add State(s) to Queue__jki_lib_state_machine.vi"("State(s) in (\"\")"=w226, "State(s) at Back (\"\")"="Setup:AxisParams\nSetup:RBSetup" ("State(s) at Back (\"\")")) -> ("States Out"=w225:string)  [unwired: 13 in]
          }
          event "MOVE MASTER": Value Change {
            n84 = event-data() -> ("NewVal"=w233:bool)  [unwired: 1 in, 5 out]
            n85 = case shown="True" w233 {
              tunnel: w232 -> [w238 w244]
              tunnel: w231 -> [w239 w243]
              tunnel: [w239 w242] -> w230
              tunnel: [w237 w241] -> w229
              frame False {
                n86 = Unbundle By Name(w238) -> ("VISA resource name"=w237:refnum<visa-resource-name>)
              }
              frame True {
                n87 = Unbundle By Name(w244) -> ("Group Cluster.Grouped?"=w245:bool)
                n88 = case shown="False" w245 {
                  tunnel: [w246 w261] -> w241
                  tunnel: w243 -> [w251 w259]
                  tunnel: [w250 w258] -> w242
                  tunnel: w244 -> [w252 w257]
                  tunnel: "MaxMotion" -> [w248 w256]
                  frame False {
                    n89 = Unbundle By Name(w252) -> ("VISA resource name"=w247:refnum<visa-resource-name>, "Master Axis"=w249:i32)
                    n90 = call <instrlib>:"Move Relative.vi"("error in (no error)"=w251, "Position (0 units)"=w248, "Axis (1)"=w249, "VISA resource name"=w247) -> ("error out"=w250:errorcluster, "VISA resource name out"=w246:refnum<visa-resource-name>)  [unwired: 2 in]
                  }
                  frame True {
                    n91 = Unbundle By Name(w257) -> ("VISA resource name"=w262:refnum<visa-resource-name>, "Master Axis"=w254:i32, "Slave Axis"=w253:i32, "Group Cluster"=w255:T10)
                    n92 = property on="Reduction Ratio (0)" class="DigNum (strict)"() -> ("Value"=w260:dbl)  [unwired: 2 in, 2 out]
                    n93 = call "ESP301GroupMove.vi"("VISA resource name"=w262, "Slave Axis"=w253, "Group Cluster"=w255, "MaxMotion"=w256, "Master Axis"=w254, "error in"=w259, "Reduction"=w260) -> ("VISA resource name out"=w261:refnum<visa-resource-name>, "error out"=w258:errorcluster)  [unwired: 7 in]
                  }
                }
              }
            }
            n94 = call <vilib>:"Add State(s) to Queue__jki_lib_state_machine.vi"("State(s) in (\"\")"=w235) -> ("States Out"=w236:string)  [unwired: 14 in]
            n95 = Bundle By Name(cluster=w232, "VISA resource name"=w229) -> (w234:T11)
          }
          event "Group Mode": Value Change {
            n96 = event-data() -> ("NewVal"=w266:bool)  [unwired: 1 in, 5 out]
            n97 = case shown="False" w266 {
              tunnel: [FALSE ("Group Cluster.Grouped?") TRUE ("Group Cluster.Grouped?")] -> w265
              tunnel: ["Setup:MotorONOFF>>OFF\nConnection:Errorcheck\nSetup:Wait>>50\nSetup:Groups>>Ungroup\nConnection:Errorcheck\nSetup:MasterSlave\nConnection:Errorcheck\nSetup:Speed\nConnection:Errorcheck\nSetup:MotorONOFF>>ON\nConnection:Errorcheck\nSetup:RBMotorPower" ("State(s) at Back (\"\")") "Setup:ReleaseMasterSlave\nSetup:Groups>>Group\nSetup:GroupSpeed\nSetup:RBGroup" ("State(s) at Back (\"\")")] -> w264
              frame False {
              }
              frame True {
              }
            }
            n98 = Bundle By Name(cluster=w267, "Group Cluster.Grouped?"=w265) -> (w268:T11)
            n99 = call <vilib>:"Add State(s) to Queue__jki_lib_state_machine.vi"("State(s) in (\"\")"=w269, "State(s) at Back (\"\")"=w264) -> ("States Out"=w270:string)  [unwired: 13 in]
          }
          event "Group Move Comp": Value Change {
            n100 = event-data() -> ()  [unwired: 1 in, 6 out]
            n101 = Unbundle By Name(w283) -> ("VISA resource name"=w282:refnum<visa-resource-name>, "Master Axis"=w278:i32, "Slave Axis"=w277:i32, "Group Cluster"=w280:T10)
            n102 = control-ref of="E Stop"() -> (w284:refnum<vi>)
            n103 = call "Comp_Group_Motion.vi"("stop 2"=w284, "Slave Axis"=w277, "Master Axis"=w278, "error in (no error)"=w276, "Motionphase"="Motionphase 2", "Group Cluster"=w280, "VISA resource name in"=w282) -> ("error out"=w275:errorcluster, "VISA resource name out"=w281:refnum<visa-resource-name>)  [unwired: 3 in]
            n104 = Bundle By Name(cluster=w283, "VISA resource name"=w281) -> (w285:T11)
            n105 = call <vilib>:"Add State(s) to Queue__jki_lib_state_machine.vi"("State(s) in (\"\")"=w286) -> ("States Out"=w287:string)  [unwired: 14 in]
          }
          event "Power Status": Value Change {
            n106 = event-data() -> ("NewVal"=w290:bool)  [unwired: 1 in, 5 out]
            n107 = Unbundle By Name(w300) -> ("VISA resource name"=w293:refnum<visa-resource-name>, "Master Axis"=w298:i32, "Slave Axis"=w297:i32)
            n108 = Build Array(w298, w297) -> (w296:i32[])
            n109 = Sort 1D Array(array=w296) -> (sorted array=w295:i32[])
            n110 = Index Array(array=w295, index=0) -> (element=w291:i32)
            n111 = call <instrlib>:"Enable Disable Motor.vi"("error in (no error)"=w289, "Action (OFF)"=w290, "Axis (1)"=w291, "VISA resource name"=w293) -> ("error out"=w288:errorcluster, "VISA resource name out"=w292:refnum<visa-resource-name>)  [unwired: 2 in]
            n112 = Bundle By Name(cluster=w300, "VISA resource name"=w292) -> (w299:T11)
            n113 = call <vilib>:"Add State(s) to Queue__jki_lib_state_machine.vi"("State(s) in (\"\")"=w302, "State(s) at Back (\"\")"="Setup:RBMotorPower" ("State(s) at Back (\"\")")) -> ("States Out"=w303:string)  [unwired: 13 in]
          }
          event "Power Status 2": Value Change {
            n114 = event-data() -> ("NewVal"=w306:bool)  [unwired: 1 in, 5 out]
            n115 = Unbundle By Name(w316) -> ("VISA resource name"=w309:refnum<visa-resource-name>, "Master Axis"=w314:i32, "Slave Axis"=w313:i32)
            n116 = Build Array(w314, w313) -> (w312:i32[])
            n117 = Sort 1D Array(array=w312) -> (sorted array=w311:i32[])
            n118 = Index Array(array=w311, index=1) -> (element=w307:i32)
            n119 = call <instrlib>:"Enable Disable Motor.vi"("error in (no error)"=w305, "Action (OFF)"=w306, "Axis (1)"=w307, "VISA resource name"=w309) -> ("error out"=w304:errorcluster, "VISA resource name out"=w308:refnum<visa-resource-name>)  [unwired: 2 in]
            n120 = Bundle By Name(cluster=w316, "VISA resource name"=w308) -> (w315:T11)
            n121 = call <vilib>:"Add State(s) to Queue__jki_lib_state_machine.vi"("State(s) in (\"\")"=w318, "State(s) at Back (\"\")"="Setup:RBMotorPower" ("State(s) at Back (\"\")")) -> ("States Out"=w319:string)  [unwired: 13 in]
          }
          event "Go steps": Value Change {
            n122 = event-data() -> ("NewVal"=w320:bool)  [unwired: 1 in, 5 out]
            n123 = case shown="True" w320 {
              tunnel: w324 -> [w329 w337]
              tunnel: [w328 w348] -> w323
              tunnel: w322 -> [w330 w345]
              tunnel: [w330 w333] -> w321
              frame False {
                n124 = Bundle By Name(cluster=w329, "Stepper Cluster.Stepped Motion"=FALSE) -> (w328:T11)
              }
              frame True {
                n125 = Unbundle By Name(w337) -> ("VISA resource name"=w347:refnum<visa-resource-name>, "Master Axis"=w332:i32, "Slave Axis"=w346:i32, "actual Position"=w331:dbl)  [unwired: 1 out]
                n126 = call <instrlib>:"Set Master-Slave Reduction Ratio.vi"("error in (no error)"=w345, "Reduction Ratio (0)"=1.0, "Axis (1)"=w346, "VISA resource name"=w347) -> ("error out"=w339:errorcluster, "VISA resource name out"=w341:refnum<visa-resource-name>)  [unwired: 2 in]
                n127 = property on="MaxMotion" class="DigNum (strict)"(error in=w339) -> (error out=w338:errorcluster, "Value"=w342:dbl)  [unwired: 1 in, 1 out]
                n128 = Tick Count (ms)() -> (millisecond timer value=w335:u32)
                n129 = call <instrlib>:"Move Relative.vi"("error in (no error)"=w338, "Position (0 units)"=w342, "Axis (1)"=w332, "VISA resource name"=w341) -> ("error out"=w333:errorcluster, "VISA resource name out"=w343:refnum<visa-resource-name>)  [unwired: 2 in]
                n130 = Bundle By Name(cluster=w337, "Stepper Cluster.Stepped Motion"=TRUE, "VISA resource name"=w343, "Stepper Cluster.act. Step"=u32 0 ("millisecond timer value"), "Stepper Cluster.millisecond timer value"=w335, "Stepper Cluster.Moving"=FALSE, "Last Position"=w331) -> (w348:T11)
              }
            }
            n131 = call <vilib>:"Add State(s) to Queue__jki_lib_state_machine.vi"("State(s) in (\"\")"=w325) -> ("States Out"=w326:string)  [unwired: 14 in]
          }
          event "Go steps 2": Value Change {
            n132 = event-data() -> ("NewVal"=w349:bool)  [unwired: 1 in, 5 out]
            n133 = case shown="True" w349 {
              tunnel: w353 -> [w358 w366]
              tunnel: [w357 w377] -> w352
              tunnel: w351 -> [w359 w374]
              tunnel: [w359 w362] -> w350
              frame False {
                n134 = Bundle By Name(cluster=w358, "Stepper Cluster 2.Stepped Motion"=FALSE ("Stepper Cluster.Stepped Motion")) -> (w357:T11)
              }
              frame True {
                n135 = Unbundle By Name(w366) -> ("VISA resource name"=w376:refnum<visa-resource-name>, "Master Axis"=w361:i32, "Slave Axis"=w375:i32, "actual Position"=w360:dbl)  [unwired: 1 out]
                n136 = call <instrlib>:"Set Master-Slave Reduction Ratio.vi"("error in (no error)"=w374, "Reduction Ratio (0)"=1.0, "Axis (1)"=w375, "VISA resource name"=w376) -> ("error out"=w368:errorcluster, "VISA resource name out"=w370:refnum<visa-resource-name>)  [unwired: 2 in]
                n137 = property on="MaxMotion" class="DigNum (strict)"(error in=w368) -> (error out=w367:errorcluster, "Value"=w371:dbl)  [unwired: 1 in, 1 out]
                n138 = Tick Count (ms)() -> (millisecond timer value=w364:u32)
                n139 = call <instrlib>:"Move Relative.vi"("error in (no error)"=w367, "Position (0 units)"=w371, "Axis (1)"=w361, "VISA resource name"=w370) -> ("error out"=w362:errorcluster, "VISA resource name out"=w372:refnum<visa-resource-name>)  [unwired: 2 in]
                n140 = Bundle By Name(cluster=w366, "Stepper Cluster 2.Stepped Motion"=TRUE ("Stepper Cluster.Stepped Motion"), "VISA resource name"=w372, "Stepper Cluster 2.act. Step"=u32 0 ("millisecond timer value"), "Stepper Cluster 2.millisecond timer value"=w364, "Stepper Cluster 2.Moving"=FALSE ("Stepper Cluster.Moving"), "Last Position"=w360) -> (w377:T11)
              }
            }
            n141 = call <vilib>:"Add State(s) to Queue__jki_lib_state_machine.vi"("State(s) in (\"\")"=w354) -> ("States Out"=w355:string)  [unwired: 14 in]
          }
          event "Go steps 3": Value Change {
            n142 = event-data() -> ("NewVal"=w378:bool)  [unwired: 1 in, 5 out]
            n143 = case shown="True" w378 {
              tunnel: w382 -> [w387 w402]
              tunnel: [w386 w403] -> w381
              tunnel: w380 -> [w388 w391]
              tunnel: [w388 w390] -> w379
              frame False {
                n144 = Bundle By Name(cluster=w387, "Stepper Cluster 3.Stepped Motion"=FALSE ("Stepper Cluster.Stepped Motion")) -> (w386:T11)
              }
              frame True {
                n145 = Unbundle By Name(w402) -> ("VISA resource name"=w400:refnum<visa-resource-name>, "Master Axis"=w398:i32, "Slave Axis"=w399:i32, "Group Cluster"=w401:T10, "actual Position"=w389:dbl)  [unwired: 1 out]
                n146 = disable-structure shown="Enabled" {
                  disable-tunnel: w401 -> [w412 _]
                  disable-tunnel: w400 -> [w411 w414]
                  disable-tunnel: w399 -> [w410 _]
                  disable-tunnel: w398 -> [w409 _]
                  disable-tunnel: "1st Holdmove" -> [w408 _]
                  disable-tunnel: [w407 w414] -> w396
                  disable-tunnel: w391 -> [w405 w413]
                  disable-tunnel: [w404 w413] -> w390
                  frame Disabled {
                    n147 = call "ESP301GroupMove.vi"("VISA resource name"=w411, "Slave Axis"=w410, "Group Cluster"=w412, "MaxMotion"=w408, "Master Axis"=w409, "error in"=w405, "Reduction"=1.0) -> ("VISA resource name out"=w407:refnum<visa-resource-name>, "error out"=w404:errorcluster)  [unwired: 7 in]
                  }
                  frame Enabled {
                  }
                }
                n148 = Tick Count (ms)() -> (millisecond timer value=w394:u32)
                n149 = Bundle By Name(cluster=w402, "Stepper Cluster 3.Stepped Motion"=TRUE, "VISA resource name"=w396, "Stepper Cluster 3.act. Step"=u32 0, "Stepper Cluster 3.millisecond timer value"=w394, "Stepper Cluster 3.Moving"=FALSE, "Last Position"=w389) -> (w403:T11)
              }
            }
            n150 = call <vilib>:"Add State(s) to Queue__jki_lib_state_machine.vi"("State(s) in (\"\")"=w383) -> ("States Out"=w384:string)  [unwired: 14 in]
          }
        }
      }
      frame "---------- Core ----------" {
        # "Do not put any code in this frame.\n(it is a separator no-op)"
        n151 = call <vilib>:"Add State(s) to Queue__jki_lib_state_machine.vi"("State(s) in (\"\")"=w418) -> ("States Out"=w417:string)  [unwired: 14 in]
      }
      frame Default {
        w428 = 42 items=["No error", "Argument error", "Memory is full", "Out of zone", "End of file", "File already open", "Generic file I/O error", "File not found", "File permission error", "Disk is full", "Duplicate path", "Too many files open", "System feature not enabled", "Resource file not found", "Cannot add resource", "Resource not found", "Image not found", "Image memory error", "Pen does not exist", "Config type invalid", "Config token not found", "Config parse error", "Config memory error", "Bad external code format", "Bad external code offset", "External code not present", "Null window", "Destroy window error", "Null menu", "Print aborted", "Bad print record", "Print driver error", "Windows error during printing", "Memory error during printing", "Print dialog error", "Generic print error", "Invalid device refnum", "Device not found", "Device parameter error", "Device unit error", "Cannot open device", "Device call aborted", "Generic error", "Cancelled by user", "Object ID too low", "Object ID too high", "Object not in heap", "Unknown heap", "Unknown object (invalid DefProc)", "Unknown object (DefProc not in table)", "Message out of range", "Invalid (null) method", "Unknown message", "Manager call not supported", "Bad address", "Network operation in progress", "Network operation timed out", "Connection is busy", "Network attribute not supported", "Network error", "Address in use", "System out of memory", "Connection aborted", "Connection refused", "Not connected", "Already connected", "Connection closed", "Initialization error (interapplication manager)", "Bad occurrence", "Wait on unbound occurrence handler", "Occurrence queue overflow", "Datalog type conflict", "Unused", "Unrecognized type (interapplication manager)", "Memory corrupt", "Failed to make temporary DLL", "Old CIN version", "Drag socket not found", "Failed to load drop-object", "Failed to register OLE object", "Failed to release OLE object", "Format specifier type mismatch", "Unknown format specifier", "Too few format specifiers", "Too many format specifiers", "Scan failed", "Newer CIN version", "Error converting to variant", "Runtime menu error", "Password tampered", "Variant attribute not found", "Incompatible variant data type", "Event data is not available", "Event Store is not present", "Occurrence is not found", "Event Queue is not created", "Event info is not available", "Refnum passed is NULL", "Error retrieving Class GUID", "Error retrieving CoClass GUID", "Error retrieving TypeLib GUID.", "Bad built application magic bytes.", "Specific driver is different from the specific driver associated with the Logical Name.", "There is no session opened to the class driver.", "Max Error", "MAX - Error with config objects", "MAX - Error loading configuration", "MAX - Group not supported"]
        # "Current State"
        # "Do not delete, rename, or modify this frame.\n(this is used to capture unhandled states and typos)"
        # "Handle mistyped state name (developer tool)"
        n152 = Format Into String(format string="Software Exception: Unhandled State \"%s\"." ("message"), error in=w424, w419) -> (resulting string=w427:string, error out=w426:errorcluster)  [unwired: 1 in]
        n153 = call <vilib>:"Error Cluster From Error Code.vi"("show call chain? (False)"=TRUE, "error in (no error)"=w426, "error message (\"\")"=w427, "error code (0)"=w428) -> ("error out"=w425:errorcluster)  [unwired: 5 in]
        n154 = call <vilib>:"Add State(s) to Queue__jki_lib_state_machine.vi"("State(s) in (\"\")"=w423) -> ("States Out"=w422:string)  [unwired: 14 in]
      }
      frame "Initialize Core Data" {
        # "Do not delete, rename, or modify this frame.\n(this is used to determine panel behavior on exit)"
        # "originally closed?"
        # "exe?"
        # "If panel starts closed or is an EXE, then close it when we exit"
        n155 = property class="VI"() -> ("Front Panel.Open"=w437:bool)  [unwired: 2 in, 2 out]
        n156 = control-ref of="Current VI Reference"() -> (w430:refnum<vi>)
        n157 = property class="App"() -> ("App.Kind"=w436:T7)  [unwired: 2 in, 2 out]
        n158 = Not(x=w437) -> (.not. x?=w434:bool)
        n159 = Equal?(x=w436, y=T7."Run Time System" ("Application:Kind")) -> (x = y?=w433:bool)
        n160 = Or(x=w434, y=w433) -> (x .or. y?=w431:bool)
        n161 = Bundle By Name(cluster=w432, "Core.Current VI Reference"=w430, "Core.Close Panel on Exit?"=w431) -> (w439:T11)
        n162 = call <vilib>:"Add State(s) to Queue__jki_lib_state_machine.vi"("State(s) in (\"\")"=w441) -> ("States Out"=w440:string)  [unwired: 14 in]
      }
      frame "Error Handler" {
        w442 = T12 2 items=["no dialog", "OK message", "continue or stop message", "OK message + warnings", "continue/stop + warnings"] ("type of dialog (OK msg:1)")
        # "Unhandled Error -- Display it"
        # "Handle any errors here.\nYou can also output any states to clean-up after errors occur"
        # "Clear error"
        n163 = call <vilib>:"General Error Handler.vi"("type of dialog (OK msg:1)"=w442, "error in (no error)"=w444) -> ()  [unwired: 9 in, 5 out]
        n164 = call <vilib>:"Add State(s) to Queue__jki_lib_state_machine.vi"("State(s) in Front (\"\")"="/* Post Error States", "State(s) in (\"\")"=w448) -> ("States Out"=w447:string)  [unwired: 13 in]
      }
      frame "Exit" {
        # "Do not put any code in this frame.\n(No errors that occur here will be handled.)"
        n165 = call <vilib>:"Add State(s) to Queue__jki_lib_state_machine.vi"("State(s) in (\"\")"=w453) -> ("States Out"=w452:string)  [unwired: 14 in]
      }
      frame "---------- Data ----------" {
        # "Do not put any code in this frame.\n(It is a separator no-op. You can make a copy of this frame to create a new Data frame)"
        n166 = call <vilib>:"Add State(s) to Queue__jki_lib_state_machine.vi"("State(s) in (\"\")"=w457) -> ("States Out"=w456:string)  [unwired: 14 in]
      }
      frame "Data: Initialize" {
        w458 = 0.0  # Last Position
        w459 = 0.0  # actual Position
        w460 = T13 {"Stepped Motion"=FALSE, "Moving"=FALSE, "millisecond timer value"=0, "act. Step"=0}  # Stepper Cluster 4
        w461 = T13 {"Stepped Motion"=FALSE, "Moving"=FALSE, "millisecond timer value"=0, "act. Step"=0}  # Stepper Cluster 3
        w462 = T10 {"Grouped?"=FALSE, "Master Axis"=0, "Group Number (1)"=0}  # Group Cluster
        w463 = T13 {"Stepped Motion"=FALSE, "Moving"=FALSE, "millisecond timer value"=0, "act. Step"=0}  # Stepper Cluster 2
        w464 = T13 {"Stepped Motion"=FALSE, "Moving"=FALSE, "millisecond timer value"=0, "act. Step"=0}  # Stepper Cluster
        w465 = FALSE  # In Motion?
        w470 = FALSE  # Connected?
        w471 = 0.0  # Acceleration (0 units/s²)
        w472 = 0.0  # Velocity (units/s)
        w473 = T14 {"Current VI Reference"=refnum, "Close Panel on Exit?"=FALSE}  # Core
        # "do not delete - used by framework"
        # "Data names and types of shift register data are defined by this bundle."
        # "Initialize the shift-register data, here.\n(data names are defined by what you wire into the bundle function)"
        n167 = Unbundle By Name("Cluster") -> ("Master Axis"=w467:i32, "Slave Axis"=w466:i32)
        n168 = Bundle("Core"=w473, "VISA resource name"=refnum<visa-resource-name> "COM1", "Velocity (units/s)"=w472, "Acceleration (0 units/s²)"=w471, "Connected?"=w470, "Master Axis"=w467, "Slave Axis"=w466, "In Motion?"=w465, "Stepper Cluster"=w464, "Stepper Cluster 2"=w463, "Group Cluster"=w462, "Stepper Cluster 3"=w461, "Stepper Cluster 4"=w460, "actual Position"=w459, "Last Position"=w458) -> (w475:T11)  [unwired: 1 in]
        n169 = call <vilib>:"Add State(s) to Queue__jki_lib_state_machine.vi"("State(s) in (\"\")"=w477) -> ("States Out"=w476:string)  [unwired: 14 in]
      }
      frame "Data: Cleanup" {
        # "Cleanup any data and references, here.\n(this is called automatically, by the Macro: Exit)"
        n170 = Unbundle By Name(w479) -> ("Core.Current VI Reference"=w481:refnum<vi>)
        n171 = Close Reference(reference=w481, error in (no error)=w478) -> (error out=w480:errorcluster)
        n172 = call <vilib>:"Add State(s) to Queue__jki_lib_state_machine.vi"("State(s) in (\"\")"=w483) -> ("States Out"=w482:string)  [unwired: 14 in]
      }
      frame "---------- UI ----------" {
        # "Do not put any code in this frame.\n(It is a separator no-op. You can make a copy of this frame to create a new UI frame)"
        n173 = call <vilib>:"Add State(s) to Queue__jki_lib_state_machine.vi"("State(s) in (\"\")"=w487) -> ("States Out"=w486:string)  [unwired: 14 in]
      }
      frame "UI: Initialize" {
        w492 = FALSE ("Serial Settings:Is Port Connected")
        w503 = "Axis"
        # "Initialize the User Interface, here.\n(this is called automatically, by the Macro: Init)"
        n174 = Unbundle By Name(w494) -> ("VISA resource name"=w489:refnum<visa-resource-name>, "Master Axis"=w497:i32, "Slave Axis"=w502:i32)
        n175 = Number To Decimal String(number=w497) -> (decimal integer string=w506:string)  [unwired: 1 in]
        n176 = Number To Decimal String(number=w502) -> (decimal integer string=w504:string)  [unwired: 1 in]
        n177 = Concatenate Strings(w503, w506) -> (w505:string)
        n178 = Concatenate Strings(w503, w504) -> (w501:string)
        n179 = Bundle(w505, "Master Axis"=w497) -> (w500:cluster{string, "Master Axis":i32})  [unwired: 1 in]
        n180 = Bundle(w501, "Slave Axis"=w502) -> (w499:cluster{string, "Slave Axis":i32})  [unwired: 1 in]
        n181 = Build Array(w500, w499) -> (w498:cluster{string, "Slave Axis":i32}[])
        n182 = property on="AXIS" class="Ring (strict)"(error in=w496, "StringsAndValues[]"=w498) -> (error out=w491:errorcluster)  [unwired: 1 in, 1 out]
        n183 = VISA Close(VISA resource name=w489, error in (no error)=w491) -> (error out=w490:errorcluster)
        n184 = Bundle By Name(cluster=w494, "Connected?"=w492, "Group Cluster.Group Number (1)"=1) -> (w493:T11)
        n185 = property on="AXIS" class="Ring (strict)"(error in=w490, "Value"=w497) -> (error out=w495:errorcluster)  [unwired: 1 in, 1 out]
        n186 = property on="Connected?" class="Bool (strict)"("Value"=w492) -> ()  [unwired: 2 in, 2 out]
        n187 = property on="Connect" class="Bool (strict)"("Value"=w492) -> ()  [unwired: 2 in, 2 out]
        n188 = call <vilib>:"Add State(s) to Queue__jki_lib_state_machine.vi"("State(s) in (\"\")"=w508) -> ("States Out"=w507:string)  [unwired: 14 in]
      }
      frame "UI: Cursor Set" {
        # "Argument"
        # "Set and Unset Cursor Busy.\n(Usage: \"UI: Cursor Set >> Busy|Idle\")"
        n189 = case shown="\"Idle\", Default" w509 {
          tunnel: w511 -> [w516 w518]
          tunnel: [w515 w517] -> w510
          frame "Idle", Default {
            n190 = call <vilib>:"Unset Busy.vi"("error in (no error)"=w516) -> ("error out"=w515:errorcluster)  [unwired: 10 in]
          }
          frame "Busy" {
            n191 = call <vilib>:"Set Busy.vi"("error in (no error)"=w518) -> ("error out"=w517:errorcluster)  [unwired: 9 in, 1 out]
          }
        }
        n192 = call <vilib>:"Add State(s) to Queue__jki_lib_state_machine.vi"("State(s) in (\"\")"=w514) -> ("States Out"=w513:string)  [unwired: 14 in]
      }
      frame "UI: Front Panel State" {
        # "Argument"
        # "Set Front Panel Open or Closed\n(Usage: \"UI: Front Panel State >> Open|Close\")"
        n193 = Unbundle By Name(w521) -> ("Core.Current VI Reference"=w520:refnum<vi>)
        n194 = case shown="\"Open\", Default" w519 {
          tunnel: w523 -> [w529 w542]
          tunnel: [w531 w543] -> w522
          tunnel: w520 -> [w530 w540]
          frame "Open", Default {
            n195 = property class="VI"(reference=w530, error in=w529) -> (reference out=w527:refnum<vi>, error out=w528:errorcluster, "Front Panel.Open"=w526:bool)
            n196 = case shown="False" w526 {
              tunnel: [w534 w537] -> w531
              tunnel: w528 -> [w533 w537]
              tunnel: w527 -> [w532 _]
              frame False {
                n197 = invoke class="VI" method="FP.Open"(reference=w532, error in=w533, "Activate"=TRUE, "State"=T8."Standard") -> (error out=w534:errorcluster)  [unwired: 1 in, 4 out]
              }
              frame True {
              }
            }
          }
          frame "Close" {
            n198 = property class="VI"(reference=w540, error in=w542) -> (reference out=w539:refnum<vi>, error out=w541:errorcluster, "Front Panel.Open"=w538:bool)
            n199 = case shown="True" w538 {
              tunnel: [w544 w547] -> w543
              tunnel: w541 -> [w544 w546]
              tunnel: w539 -> [_ w545]
              frame False {
              }
              frame True {
                n200 = invoke class="VI" method="FP.Close"(reference=w545, error in=w546) -> (error out=w547:errorcluster)  [unwired: 1 in, 2 out]
              }
            }
          }
        }
        n201 = call <vilib>:"Add State(s) to Queue__jki_lib_state_machine.vi"("State(s) in (\"\")"=w525) -> ("States Out"=w524:string)  [unwired: 14 in]
      }
      frame "---------- Macro ----------" {
        # "Do not put any code in this frame.\n(It is a separator no-op. You can make a copy of this frame to create a new Macro frame)"
        n202 = call <vilib>:"Add State(s) to Queue__jki_lib_state_machine.vi"("State(s) in (\"\")"=w551) -> ("States Out"=w550:string)  [unwired: 14 in]
      }
      frame "Macro: Initialize" {
        w552 = "Data: Initialize\nInitialize Core Data\nUI: Initialize\nUI: Front Panel State >> Open"  # Data: Initialize Initialize Core Data UI: Initialize UI: Front Panel State >> Open
        # "Initialization Macro\n(This is called once, when the VI starts)"
        n203 = call <vilib>:"Add State(s) to Queue__jki_lib_state_machine.vi"("State(s) in Front (\"\")"=w552, "State(s) in (\"\")"=w556) -> ("States Out"=w555:string)  [unwired: 13 in]
      }
      frame "Macro: Exit" {
        # "Exit Macro\n(This is called once, when the VI exits)"
        n204 = Unbundle By Name(w570) -> ("Core.Close Panel on Exit?"=w569:bool, "Connected?"=w562:bool)
        n205 = Select(t="Setup:KillGroups\nConnection:Close", s=w562, f="") -> (s? t:f=w560:string)
        n206 = Concatenate Strings("Data: Cleanup\n", w560, "\n", "Exit" ("string")) -> (w563:string)
        n207 = Select(t="UI: Front Panel State >> Close", s=w569, f="") -> (s? t:f=w566:string)
        n208 = call <vilib>:"Add State(s) to Queue__jki_lib_state_machine.vi"("State(s) in (\"\")"=w566, "State(s) at Back (\"\")"=w563) -> ("States Out"=w565:string)  [unwired: 13 in]
        n209 = call <vilib>:"Add State(s) to Queue__jki_lib_state_machine.vi"("State(s) in Front (\"\")"=w565, "State(s) in (\"\")"=w573) -> ("States Out"=w572:string)  [unwired: 13 in]
      }
      frame "----------Setup ----------" {
        # "Template Separator\n(You can make a copy of, or modify, this frame)"
        n210 = call <vilib>:"Add State(s) to Queue__jki_lib_state_machine.vi"("State(s) in (\"\")"=w577) -> ("States Out"=w576:string)  [unwired: 14 in]
      }
      frame "Setup:MotorONOFF" {
        # "Template Separator\n(You can make a copy of, or modify, this frame)"
        n211 = Unbundle By Name(w587) -> ("VISA resource name"=w582:refnum<visa-resource-name>, "Master Axis"=w585:i32, "Slave Axis"=w584:i32)
        n212 = case shown="\"ON\"" w583 {
          tunnel: [FALSE ("Action (OFF)") TRUE ("Action (OFF)")] -> w578
          frame "OFF", Default {
          }
          frame "ON" {
          }
        }
        n213 = call <instrlib>:"Enable Disable Motor.vi"("error in (no error)"=w580, "Action (OFF)"=w578, "Axis (1)"=w585, "VISA resource name"=w582) -> ("error out"=w589:errorcluster, "VISA resource name out"=w588:refnum<visa-resource-name>)  [unwired: 2 in]
        n214 = call <instrlib>:"Enable Disable Motor.vi"("error in (no error)"=w589, "Action (OFF)"=w578, "Axis (1)"=w584, "VISA resource name"=w588) -> ("error out"=w579:errorcluster, "VISA resource name out"=w581:refnum<visa-resource-name>)  [unwired: 2 in]
        n215 = Bundle By Name(cluster=w587, "VISA resource name"=w581) -> (w586:T11)
        n216 = call <vilib>:"Add State(s) to Queue__jki_lib_state_machine.vi"("State(s) in (\"\")"=w591) -> ("States Out"=w590:string)  [unwired: 14 in]
      }
      frame "Setup:SlaveOFF" {
        # "Template Separator\n(You can make a copy of, or modify, this frame)"
        n217 = Unbundle By Name(w601) -> ("VISA resource name"=w594:refnum<visa-resource-name>, "Slave Axis"=w599:i32)  [unwired: 1 out]
        n218 = call <instrlib>:"Enable Disable Motor.vi"("error in (no error)"=w596, "Action (OFF)"=FALSE, "Axis (1)"=w599, "VISA resource name"=w594) -> ("error out"=w597:errorcluster, "VISA resource name out"=w598:refnum<visa-resource-name>)  [unwired: 2 in]
        n219 = Bundle By Name(cluster=w601, "VISA resource name"=w598) -> (w600:T11)
        n220 = call <vilib>:"Add State(s) to Queue__jki_lib_state_machine.vi"("State(s) in (\"\")"=w603) -> ("States Out"=w602:string)  [unwired: 14 in]
      }
      frame "Setup:RBMotorPower" {
        # "Template Separator\n(You can make a copy of, or modify, this frame)"
        n221 = Unbundle By Name(w619) -> ("VISA resource name"=w611:refnum<visa-resource-name>, "Master Axis"=w616:i32, "Slave Axis"=w615:i32)
        n222 = Build Array(w616, w615) -> (w614:i32[])
        n223 = Sort 1D Array(array=w614) -> (sorted array=w613:i32[])
        n224 = for {
          tunnel: w611 -> [w627]
          tunnel: w617 -> [w626]
          tunnel: w613 -> [w625] mode=indexing
          tunnel: [w622] -> w612 mode=indexing
          tunnel: [w624] -> w610 mode=indexing
          tunnel: [w623] -> w608
          n225 = call <instrlib>:"Get Motor Power Status.vi"("error in (no error)"=w626, "Axis (1)"=w625, "VISA resource name"=w627) -> ("error out"=w624:errorcluster, "Power Status"=w622:bool, "VISA resource name out"=w623:refnum<visa-resource-name>)  [unwired: 2 in]
        }
        n226 = Merge Errors(w610) -> (w609:errorcluster)
        n227 = Bundle By Name(cluster=w619, "VISA resource name"=w608) -> (w618:T11)
        n228 = Index Array(array=w612, index #1=0 ("index"), index #2=1 ("index")) -> (element #1=w605:bool, element #2=w604:bool)
        n229 = property on="Power Status" class="Bool (strict)"("Value"=w605) -> ()  [unwired: 2 in, 2 out]
        n230 = property on="Power Status 2" class="Bool (strict)"("Value"=w604) -> ()  [unwired: 2 in, 2 out]
        n231 = call <vilib>:"Add State(s) to Queue__jki_lib_state_machine.vi"("State(s) in (\"\")"=w621) -> ("States Out"=w620:string)  [unwired: 14 in]
      }
      frame "Setup:Wait" {
        # "Template Separator\n(You can make a copy of, or modify, this frame)"
        n232 = Decimal String To Number(string=w630) -> (number=w629:i32)  [unwired: 2 in, 1 out]
        n233 = Wait (ms)(milliseconds to wait=w629) -> ()  [unwired: 1 out]
        n234 = call <vilib>:"Add State(s) to Queue__jki_lib_state_machine.vi"("State(s) in (\"\")"=w633) -> ("States Out"=w632:string)  [unwired: 14 in]
      }
      frame "Setup:MasterSlave" {
        # "Template Separator\n(You can make a copy of, or modify, this frame)"
        n235 = Unbundle By Name(w645) -> ("VISA resource name"=w642:refnum<visa-resource-name>, "Master Axis"=w643:i32, "Slave Axis"=w638:i32)
        n236 = call <instrlib>:"Define Master Slave Relationship.vi"("error in (no error)"=w641, "Master Axis"=w643, "Slave Axis"=w638, "VISA resource name"=w642) -> ("error out"=w639:errorcluster, "VISA resource name out"=w640:refnum<visa-resource-name>)  [unwired: 2 in]
        n237 = call <instrlib>:"Set Trajectory Mode.vi"("Trajectory Mode"=T9."Slave to master's desired position (trajectory)", "error in (no error)"=w639, "Axis (1)"=w638, "VISA resource name"=w640) -> ("error out"=w635:errorcluster, "VISA resource name out"=w636:refnum<visa-resource-name>)  [unwired: 3 in]
        n238 = call <instrlib>:"Set Trajectory Mode.vi"("Trajectory Mode"=T9."Trapezoidal Mode", "error in (no error)"=w635, "Axis (1)"=w643, "VISA resource name"=w636) -> ("error out"=w634:errorcluster, "VISA resource name out"=w637:refnum<visa-resource-name>)  [unwired: 3 in]
        n239 = Bundle By Name(cluster=w645, "VISA resource name"=w637) -> (w644:T11)
        n240 = call <vilib>:"Add State(s) to Queue__jki_lib_state_machine.vi"("State(s) in (\"\")"=w649) -> ("States Out"=w648:string)  [unwired: 14 in]
      }
      frame "Setup:Groups" {
        # "Template Separator\n(You can make a copy of, or modify, this frame)"
        n241 = Unbundle By Name(w660) -> ("VISA resource name"=w658:refnum<visa-resource-name>, "Master Axis"=w653:i32, "Slave Axis"=w652:i32)
        n242 = Build Array(w653, w652) -> (w651:i32[])
        n243 = case shown="\"Ungroup\", Default" w654 {
          tunnel: w658 -> [w666 w673]
          tunnel: w657 -> [w667 w672]
          tunnel: [w664 w671] -> w656
          tunnel: [w663 w670] -> w655
          tunnel: w651 -> [_ w669]
          tunnel: 1 ("Group Number (1)") -> [w665 w668]
          frame "Ungroup", Default {
            n244 = call <instrlib>:"Delete Group.vi"("error in (no error)"=w667, "Group Number (1)"=w665, "VISA resource name"=w666) -> ("error out"=w664:errorcluster, "VISA resource name out"=w663:refnum<visa-resource-name>)  [unwired: 3 in]
          }
          frame "Group" {
            n245 = call <instrlib>:"Create A New Group.vi"("error in (no error)"=w672, "Axis Number"=w669, "Group Number (1)"=w668, "VISA resource name"=w673) -> ("error out"=w671:errorcluster, "VISA resource name out"=w670:refnum<visa-resource-name>)  [unwired: 2 in]
          }
        }
        n246 = Bundle By Name(cluster=w660, "VISA resource name"=w655) -> (w659:T11)
        n247 = call <vilib>:"Add State(s) to Queue__jki_lib_state_machine.vi"("State(s) in (\"\")"=w662) -> ("States Out"=w661:string)  [unwired: 14 in]
      }
      frame "Setup:ReleaseMasterSlave" {
        # "Template Separator\n(You can make a copy of, or modify, this frame)"
        n248 = Unbundle By Name(w681) -> ("VISA resource name"=w678:refnum<visa-resource-name>, "Master Axis"=w675:i32, "Slave Axis"=w674:i32)
        n249 = case shown="No Error" w679 {
          selector: w679 -> [w687 w698]
          tunnel: [w688 w698] -> w676
          tunnel: w678 -> [w686 w697]
          tunnel: [w689 w697] -> w677
          tunnel: w675 -> [w691 _]
          tunnel: w674 -> [w690 _]
          frame No Error {
            w694 = T9."Trapezoidal Mode" ("Trajectory Mode")
            n250 = call <instrlib>:"Set Trajectory Mode.vi"("Trajectory Mode"=w694, "error in (no error)"=w687, "Axis (1)"=w691, "VISA resource name"=w686) -> ("error out"=w696:errorcluster, "VISA resource name out"=w695:refnum<visa-resource-name>)  [unwired: 3 in]
            n251 = call <instrlib>:"Set Trajectory Mode.vi"("Trajectory Mode"=w694, "error in (no error)"=w696, "Axis (1)"=w690, "VISA resource name"=w695) -> ("error out"=w684:errorcluster, "VISA resource name out"=w685:refnum<visa-resource-name>)  [unwired: 3 in]
            n252 = call <instrlib>:"Define Master Slave Relationship.vi"("error in (no error)"=w684, "Master Axis"=w691, "Slave Axis"=w691, "VISA resource name"=w685) -> ("error out"=w693:errorcluster, "VISA resource name out"=w692:refnum<visa-resource-name>)  [unwired: 2 in]
            n253 = call <instrlib>:"Define Master Slave Relationship.vi"("error in (no error)"=w693, "Master Axis"=w690, "Slave Axis"=w690, "VISA resource name"=w692) -> ("error out"=w688:errorcluster, "VISA resource name out"=w689:refnum<visa-resource-name>)  [unwired: 2 in]
          }
          frame Error {
            (unwired) -1 ("Group Number (1)")
          }
        }
        n254 = Bundle By Name(cluster=w681, "VISA resource name"=w677) -> (w680:T11)
        n255 = call <vilib>:"Add State(s) to Queue__jki_lib_state_machine.vi"("State(s) in (\"\")"=w683) -> ("States Out"=w682:string)  [unwired: 14 in]
      }
      frame "Setup:Speed" {
        # "Your code here.\n(You can make a copy of, or modify, this frame)"
        n256 = Unbundle By Name(w715) -> ("VISA resource name"=w713:refnum<visa-resource-name>, "Slave Axis"=w702:i32)
        n257 = call <instrlib>:"Set Master-Slave Jog Velocity Update Interval.vi"("error in (no error)"=w711, "Interval"="Interval", "VISA resource name"=w713) -> ("error out"=w710:errorcluster, "VISA resource name out"=w712:refnum<visa-resource-name>)  [unwired: 3 in]
        n258 = call <instrlib>:"Set Master-Slave Reduction Ratio.vi"("error in (no error)"=w710, "Reduction Ratio (0)"="Reduction Ratio (0)", "Axis (1)"=w702, "VISA resource name"=w712) -> ("error out"=w700:errorcluster, "VISA resource name out"=w699:refnum<visa-resource-name>)  [unwired: 2 in]
        n259 = call <instrlib>:"Get Master-Slave Velocity Update Interval.vi"("error in (no error)"=w700, "VISA resource name"=w699) -> ("error out"=w706:errorcluster, "Interval (ms)"=→"Interval (ms)":i32, "VISA resource name out"=w707:refnum<visa-resource-name>)  [unwired: 3 in]
        n260 = call <instrlib>:"Get Master-Slave Reduction Ratio.vi"("error in (no error)"=w706, "Axis (1)"=w702, "VISA resource name"=w707) -> ("error out"=w703:errorcluster, "Reduction Ratio"=→"Reduction Ratio":dbl, "VISA resource name out"=w704:refnum<visa-resource-name>)  [unwired: 2 in]
        n261 = Bundle By Name(cluster=w715, "VISA resource name"=w704) -> (w714:T11)
        n262 = call <vilib>:"Add State(s) to Queue__jki_lib_state_machine.vi"("State(s) in (\"\")"=w717) -> ("States Out"=w716:string)  [unwired: 14 in]
      }
      frame "Setup:RBSetup" {
        # "Your code here.\n(You can make a copy of, or modify, this frame)"
        n263 = Unbundle By Name(w729) -> ("VISA resource name"=w724:refnum<visa-resource-name>, "Master Axis"=w721:i32, "Slave Axis"=w720:i32)  [unwired: 1 out]
        n264 = Build Array(w721, w720) -> (w719:i32[])
        n265 = Sort 1D Array(array=w719) -> (sorted array=w718:i32[])
        n266 = for {
          tunnel: w727 -> [w758]
          tunnel: [w751] -> w726 mode=indexing
          tunnel: w724 -> [w750]
          tunnel: [w744] -> w723
          tunnel: [w734] -> w722 mode=indexing
          tunnel: w718 -> [w732] mode=indexing
          n267 = call <instrlib>:"Get Maximum Acceleration and Deceleration.vi"("error in (no error)"=w758, "Axis (1)"=w732, "VISA resource name"=w750) -> ("error out"=w757:errorcluster, "Acceleration (units/s²)"=w743:dbl, "VISA resource name out"=w749:refnum<visa-resource-name>)  [unwired: 2 in]
          n268 = call <instrlib>:"Get Maximum Velocity.vi"("error in (no error)"=w757, "Axis (1)"=w732, "VISA resource name"=w749) -> ("error out"=w756:errorcluster, "Maximum Velocity (units/s)"=w742:dbl, "VISA resource name out"=w748:refnum<visa-resource-name>)  [unwired: 2 in]
          n269 = call <instrlib>:"Get Acceleration.vi"("error in (no error)"=w756, "Axis (1)"=w732, "VISA resource name"=w748) -> ("error out"=w755:errorcluster, "Acceleration (units/s²)"=w741:dbl, "VISA resource name out"=w747:refnum<visa-resource-name>)  [unwired: 2 in]
          n270 = call <instrlib>:"Get Deceleration.vi"("error in (no error)"=w755, "Axis (1)"=w732, "VISA resource name"=w747) -> ("error out"=w754:errorcluster, "Deceleration (units/s²)"=w740:dbl, "VISA resource name out"=w746:refnum<visa-resource-name>)  [unwired: 2 in]
          n271 = call <instrlib>:"Get Velocity.vi"("error in (no error)"=w754, "Axis (1)"=w732, "VISA resource name"=w746) -> ("error out"=w753:errorcluster, "Velocity (units/s)"=w733:dbl, "VISA resource name out"=w739:refnum<visa-resource-name>)  [unwired: 2 in]
          n272 = Bundle("Acceleration (units/s²)"=w743, "Maximum Velocity (units/s)"=w742, "Acceleration (units/s²)"=w741, "Deceleration (units/s²)"=w740, "Velocity (units/s)"=w733) -> (w736:T15)  [unwired: 1 in]
          n273 = call <instrlib>:"Get Acceleration Feed-Forward Gain.vi"("error in (no error)"=w753, "Axis (1)"=w732, "VISA resource name"=w739) -> ("error out"=w752:errorcluster, "Gain"=w738:dbl, "VISA resource name out"=w745:refnum<visa-resource-name>)  [unwired: 2 in]
          n274 = call <instrlib>:"Get Velocity Feed-Forward Gain.vi"("error in (no error)"=w752, "Axis (1)"=w732, "VISA resource name"=w745) -> ("error out"=w751:errorcluster, "Gain"=w737:dbl, "VISA resource name out"=w744:refnum<visa-resource-name>)  [unwired: 2 in]
          n275 = Bundle("Gain"=w738, "Gain"=w737) -> (w735:cluster{"Gain":dbl, "Gain":dbl})  [unwired: 1 in]
          n276 = Bundle(w736, w735) -> (w734:T16)  [unwired: 1 in]
        }
        "Array" <- w722
        n277 = Bundle By Name(cluster=w729, "VISA resource name"=w723) -> (w728:T11)
        n278 = Merge Errors(w726) -> (w725:errorcluster)
        n279 = call <vilib>:"Add State(s) to Queue__jki_lib_state_machine.vi"("State(s) in (\"\")"=w731) -> ("States Out"=w730:string)  [unwired: 14 in]
      }
      frame "Setup:RBFBFilter" {
        # "Your code here.\n(You can make a copy of, or modify, this frame)"
        n280 = Unbundle By Name(w770) -> ("VISA resource name"=w765:refnum<visa-resource-name>, "Master Axis"=w763:i32, "Slave Axis"=w762:i32)  [unwired: 1 out]
        n281 = Build Array(w763, w762) -> (w761:i32[])
        n282 = Sort 1D Array(array=w761) -> (sorted array=w760:i32[])
        n283 = for {
          tunnel: w768 -> [w782]
          tunnel: [w778] -> w767 mode=indexing
          tunnel: w765 -> [w788]
          tunnel: [w784] -> w764
          tunnel: [w773] -> w759 mode=indexing
          tunnel: w760 -> [w783] mode=indexing
          n284 = call <instrlib>:"Get Saturation Level Of Integral Factor.vi"("error in (no error)"=w782, "Axis (1)"=w783, "VISA resource name"=w788) -> ("error out"=w781:errorcluster, "Ks"=w776:dbl, "VISA resource name out"=w787:refnum<visa-resource-name>)  [unwired: 2 in]
          n285 = call <instrlib>:"Get proportional Gain.vi"("error in (no error)"=w781, "Axis (1)"=w783, "VISA resource name"=w787) -> ("error out"=w780:errorcluster, "Kp"=w775:dbl, "VISA resource name out"=w786:refnum<visa-resource-name>)  [unwired: 2 in]
          n286 = call <instrlib>:"Get Integral Gain.vi"("error in (no error)"=w780, "Axis (1)"=w783, "VISA resource name"=w786) -> ("error out"=w779:errorcluster, "Ki"=w774:dbl, "VISA resource name out"=w785:refnum<visa-resource-name>)  [unwired: 2 in]
          n287 = call <instrlib>:"Get Derivative Gain.vi"("error in (no error)"=w779, "Axis (1)"=w783, "VISA resource name"=w785) -> ("error out"=w778:errorcluster, "Kd"=w777:dbl, "VISA resource name out"=w784:refnum<visa-resource-name>)  [unwired: 2 in]
          n288 = Bundle("Ks"=w776, "Kp"=w775, "Ki"=w774, "Kd"=w777) -> (w773:cluster{"Ks":dbl, "Kp":dbl, "Ki":dbl, "Kd":dbl})  [unwired: 1 in]
        }
        "FilterSetup" <- w759
        n289 = Bundle By Name(cluster=w770, "VISA resource name"=w764) -> (w769:T11)
        n290 = Merge Errors(w767) -> (w766:errorcluster)
        n291 = call <vilib>:"Add State(s) to Queue__jki_lib_state_machine.vi"("State(s) in (\"\")"=w772) -> ("States Out"=w771:string)  [unwired: 14 in]
      }
      frame "Setup:InitButtons" {
        # "Your code here.\n(You can make a copy of, or modify, this frame)"
        n292 = Unbundle By Name(w817) -> ("VISA resource name"=w814:refnum<visa-resource-name>)  [unwired: 3 out]
        n293 = property on="AXIS" class="Ring (strict)"() -> ("Value"=w794:i32)  [unwired: 2 in, 2 out]
        n294 = call <instrlib>:"Get Maximum Acceleration and Deceleration.vi"("error in (no error)"=w815, "Axis (1)"=w794, "VISA resource name"=w814) -> ("error out"=w813:errorcluster, "Acceleration (units/s²)"=w801:dbl, "VISA resource name out"=w807:refnum<visa-resource-name>)  [unwired: 2 in]
        n295 = property on="Max Acceleration (0 units/s²)" class="DigNum (strict)"("Value"=w801) -> ()  [unwired: 2 in, 2 out]
        n296 = call <instrlib>:"Get Maximum Velocity.vi"("error in (no error)"=w813, "Axis (1)"=w794, "VISA resource name"=w807) -> ("error out"=w812:errorcluster, "Maximum Velocity (units/s)"=w797:dbl, "VISA resource name out"=w806:refnum<visa-resource-name>)  [unwired: 2 in]
        n297 = property on="Maximum Velocity (0 units/s)" class="DigNum (strict)"("Value"=w797) -> ()  [unwired: 2 in, 2 out]
        n298 = call <instrlib>:"Get Acceleration.vi"("error in (no error)"=w812, "Axis (1)"=w794, "VISA resource name"=w806) -> ("error out"=w811:errorcluster, "Acceleration (units/s²)"=w796:dbl, "VISA resource name out"=w805:refnum<visa-resource-name>)  [unwired: 2 in]
        n299 = call <instrlib>:"Get Deceleration.vi"("error in (no error)"=w811, "Axis (1)"=w794, "VISA resource name"=w805) -> ("error out"=w810:errorcluster, "Deceleration (units/s²)"=w795:dbl, "VISA resource name out"=w804:refnum<visa-resource-name>)  [unwired: 2 in]
        n300 = property on="Deceleration (0 units/s²)" class="DigNum (strict)"("Value"=w795) -> ()  [unwired: 2 in, 2 out]
        n301 = property on="Acceleration (0 units/s²)" class="DigNum (strict)"("Value"=w796) -> ()  [unwired: 2 in, 2 out]
        n302 = call <instrlib>:"Get Velocity.vi"("error in (no error)"=w810, "Axis (1)"=w794, "VISA resource name"=w804) -> ("error out"=w809:errorcluster, "Velocity (units/s)"=w798:dbl, "VISA resource name out"=w802:refnum<visa-resource-name>)  [unwired: 2 in]
        n303 = property on="Velocity (units/s)" class="DigNum (strict)"("Value"=w798) -> ()  [unwired: 2 in, 2 out]
        n304 = call <instrlib>:"Get Acceleration Feed-Forward Gain.vi"("error in (no error)"=w809, "Axis (1)"=w794, "VISA resource name"=w802) -> ("error out"=w808:errorcluster, "Gain"=w799:dbl, "VISA resource name out"=w803:refnum<visa-resource-name>)  [unwired: 2 in]
        n305 = call <instrlib>:"Get Velocity Feed-Forward Gain.vi"("error in (no error)"=w808, "Axis (1)"=w794, "VISA resource name"=w803) -> ("error out"=w790:errorcluster, "Gain"=w800:dbl, "VISA resource name out"=w793:refnum<visa-resource-name>)  [unwired: 2 in]
        n306 = property on="Acceleration feed-forward gain factor (0)" class="DigNum (strict)"("Value"=w799) -> ()  [unwired: 2 in, 2 out]
        n307 = property on="Velocity feed-forward gain factor (0)" class="DigNum (strict)"("Value"=w800) -> ()  [unwired: 2 in, 2 out]
        n308 = call <instrlib>:"Get DAC Offset.vi"("error in (no error)"=w790, "Axis (1)"=w794, "VISA resource name"=w793) -> ("error out"=w789:errorcluster, "DAC Offset"=w791:dbl, "VISA resource name out"=w792:refnum<visa-resource-name>)  [unwired: 2 in]
        n309 = Bundle By Name(cluster=w817, "VISA resource name"=w792) -> (w816:T11)
        n310 = property on="DAC Offset (0)" class="DigNum (strict)"("Value"=w791) -> ()  [unwired: 2 in, 2 out]
        n311 = call <vilib>:"Add State(s) to Queue__jki_lib_state_machine.vi"("State(s) in (\"\")"=w819) -> ("States Out"=w818:string)  [unwired: 14 in]
      }
      frame "Setup:PIDFilter" {
        # "Your code here.\n(You can make a copy of, or modify, this frame)"
        n312 = Unbundle By Name(w826) -> ("VISA resource name"=w824:refnum<visa-resource-name>, "Connected?"=w820:bool)
        n313 = case shown="True" w820 {
          tunnel: w824 -> [w829 w840]
          tunnel: w823 -> [w831 w839]
          tunnel: [w829 w833] -> w822
          tunnel: [w830 w832] -> w821
          frame False {
            n314 = call "Display Message to User2"("error in (no error)"=w831) -> ("error out"=w830:errorcluster)  [unwired: 9 in, 1 out]
          }
          frame True {
            n315 = call <instrlib>:"Set Acceleration Feed-Forward Gain.vi"("error in (no error)"=w839, "Acceleration feed-forward gain factor (0)"="Acceleration feed-forward gain factor (0)", "Axis (1)"="AXIS", "VISA resource name"=w840) -> ("error out"=w838:errorcluster, "VISA resource name out"=w837:refnum<visa-resource-name>)  [unwired: 2 in]
            n316 = call <instrlib>:"Set Velocity Feed-Forward Gain.vi"("error in (no error)"=w838, "Velocity feed-forward gain factor (0)"="Velocity feed-forward gain factor (0)", "Axis (1)"="AXIS", "VISA resource name"=w837) -> ("error out"=w835:errorcluster, "VISA resource name out"=w834:refnum<visa-resource-name>)  [unwired: 2 in]
            n317 = call <instrlib>:"Update Servo Filter.vi"("error in (no error)"=w835, "Axis (0)"="AXIS", "VISA resource name"=w834) -> ("error out"=w832:errorcluster, "VISA resource name out"=w833:refnum<visa-resource-name>)  [unwired: 3 in]
          }
        }
        n318 = Bundle By Name(cluster=w826, "VISA resource name"=w822) -> (w825:T11)
        n319 = call <vilib>:"Add State(s) to Queue__jki_lib_state_machine.vi"("State(s) in (\"\")"=w828) -> ("States Out"=w827:string)  [unwired: 14 in]
      }
      frame "Setup:AxisParams" {
        # "Your code here.\n(You can make a copy of, or modify, this frame)"
        n320 = Unbundle By Name(w849) -> ("VISA resource name"=w847:refnum<visa-resource-name>, "Connected?"=w843:bool)
        n321 = case shown="True" w843 {
          tunnel: w847 -> [w852 w870]
          tunnel: w846 -> [w854 w864]
          tunnel: [w852 w855] -> w845
          tunnel: [w853 w856] -> w844
          frame False {
            n322 = call "Display Message to User"("error in (no error)"=w854) -> ("error out"=w853:errorcluster)  [unwired: 9 in, 1 out]
          }
          frame True {
            n323 = property on="AXIS" class="Ring (strict)"() -> ("Value"=w857:i32)  [unwired: 2 in, 2 out]
            n324 = call <instrlib>:"Set Maximum Velocity.vi"("error in (no error)"=w864, "Maximum Velocity (0 units/s)"="Maximum Velocity (0 units/s)", "Axis (1)"=w857, "VISA resource name"=w870) -> ("error out"=w863:errorcluster, "VISA resource name out"=w867:refnum<visa-resource-name>)  [unwired: 2 in]
            n325 = call <instrlib>:"Set Maximum Acceleration and Deceleration.vi"("error in (no error)"=w863, "Acceleration (0 units/s²)"="Max Acceleration (0 units/s²)", "Axis (1)"=w857, "VISA resource name"=w867) -> ("error out"=w862:errorcluster, "VISA resource name out"=w866:refnum<visa-resource-name>)  [unwired: 2 in]
            n326 = call <instrlib>:"Set Acceleration.vi"("error in (no error)"=w862, "Acceleration (0 units/s²)"="Acceleration (0 units/s²)", "Axis (1)"=w857, "VISA resource name"=w866) -> ("error out"=w861:errorcluster, "VISA resource name out"=w865:refnum<visa-resource-name>)  [unwired: 2 in]
            n327 = call <instrlib>:"Set Deceleration.vi"("error in (no error)"=w861, "Deceleration (0 units/s²)"="Deceleration (0 units/s²)", "Axis (1)"=w857, "VISA resource name"=w865) -> ("error out"=w859:errorcluster, "VISA resource name out"=w860:refnum<visa-resource-name>)  [unwired: 2 in]
            n328 = call <instrlib>:"Set Velocity.vi"("error in (no error)"=w859, "Velocity (units/s)"="Velocity (units/s)", "Axis (1)"=w857, "VISA resource name"=w860) -> ("error out"=w856:errorcluster, "VISA resource name out"=w855:refnum<visa-resource-name>)  [unwired: 2 in]
          }
        }
        n329 = Bundle By Name(cluster=w849, "VISA resource name"=w845) -> (w848:T11)
        n330 = call <vilib>:"Add State(s) to Queue__jki_lib_state_machine.vi"("State(s) in (\"\")"=w851) -> ("States Out"=w850:string)  [unwired: 14 in]
      }
      frame "Setup:GroupSpeed" {
        # "Your code here.\n(You can make a copy of, or modify, this frame)"
        n331 = Unbundle By Name(w880) -> ("VISA resource name"=w878:refnum<visa-resource-name>, "Connected?"=w877:bool, "Group Cluster.Group Number (1)"=w874:i32)
        n332 = case shown="True" w877 {
          tunnel: w878 -> [w884 w914]
          tunnel: w876 -> [w883 w912]
          tunnel: [w884 w892] -> w875
          tunnel: w874 -> [_ w913]
          tunnel: [w883 w887] -> w873
          frame False {
            n333 = call "Display Message to User6"() -> ()  [unwired: 10 in, 2 out]
          }
          frame True {
            n334 = flat-sequence {
              tunnel: w914 -> [w920]
              tunnel: w913 -> [w915]
              tunnel: w912 -> [w919]
              tunnel: [w917] -> w911
              tunnel: [w916] -> w909
              tunnel: [w915] -> w907
              tunnel: [w915] -> w905
              tunnel: w911 -> [w925]
              tunnel: [w925] -> w910
              tunnel: w909 -> [w924]
              tunnel: [w924] -> w908
              tunnel: w907 -> [w923]
              tunnel: [w923] -> w906
              tunnel: w905 -> [w922]
              tunnel: [w922] -> w904
              tunnel: [w921] -> w903
              tunnel: "groupInit Delay" -> [w921]
              tunnel: w910 -> [w933]
              tunnel: [w932] -> w901
              tunnel: w908 -> [w931]
              tunnel: [w930] -> w899
              tunnel: w906 -> [w929]
              tunnel: [w928] -> w897
              tunnel: w904 -> [w928]
              tunnel: w903 -> [w926]
              tunnel: [w926] -> w895
              tunnel: w901 -> [w937]
              tunnel: [w937] -> w900
              tunnel: w899 -> [w936]
              tunnel: [w936] -> w898
              tunnel: w897 -> [w935]
              tunnel: [w935] -> w896
              tunnel: w895 -> [w934]
              tunnel: [w934] -> w885
              tunnel: w900 -> [w944]
              tunnel: w898 -> [w943]
              tunnel: w896 -> [w940]
              tunnel: [w941] -> w893
              tunnel: [w940] -> w891
              tunnel: [w939] -> w889
              tunnel: [w938] -> w886
              tunnel: w885 -> [w938]
              tunnel: [w948] -> w894
              tunnel: w893 -> [w948]
              tunnel: w891 -> [w947]
              tunnel: [w947] -> w890
              tunnel: w889 -> [w946]
              tunnel: [w946] -> w888
              tunnel: w886 -> [w945]
              tunnel: w894 -> [w954]
              tunnel: [w953] -> w892
              tunnel: w890 -> [w952]
              tunnel: w888 -> [w951]
              tunnel: [w950] -> w887
              frame #0 {
                n335 = call <instrlib>:"Set Group Velocity.vi"("error in (no error)"=w919, "Velocity (units/s)"="Group Velocity (units/s)", "Group Number (1)"=w915, "VISA resource name"=w920) -> ("error out"=w916:errorcluster, "VISA resource name out"=w917:refnum<visa-resource-name>)  [unwired: 2 in]
              }
              frame #1 {
                n336 = Wait (ms)(milliseconds to wait=w921) -> ()  [unwired: 1 out]
              }
              frame #2 {
                n337 = call <instrlib>:"Set Group Acceleration.vi"("error in (no error)"=w931, "Acceleration (0 units/s²)"="Group Acceleration\n (0 units/s²)", "Group Number (1)"=w929, "VISA resource name"=w933) -> ("error out"=w930:errorcluster, "VISA resource name out"=w932:refnum<visa-resource-name>)  [unwired: 2 in]
              }
              frame #3 {
                n338 = Wait (ms)(milliseconds to wait=w934) -> ()  [unwired: 1 out]
              }
              frame #4 {
                n339 = call <instrlib>:"Set Group Jerk.vi"("error in (no error)"=w943, "Vector Jerk (0 units/s^3)"="Group Vector Jerk\n (0 units/s^3)", "Group Number (1)"=w940, "VISA resource name"=w944) -> ("error out"=w939:errorcluster, "VISA resource name out"=w941:refnum<visa-resource-name>)  [unwired: 2 in]
              }
              frame #5 {
                n340 = Wait (ms)(milliseconds to wait=w945) -> ()  [unwired: 1 out]
              }
              frame #6 {
                n341 = call <instrlib>:"Set Group Decceleration.vi"("error in (no error)"=w951, "Decceleration (0 units/s²)"="Group Decceleration \n(0 units/s²)", "Group Number (1)"=w952, "VISA resource name"=w954) -> ("error out"=w950:errorcluster, "VISA resource name out"=w953:refnum<visa-resource-name>)  [unwired: 2 in]
              }
            }
          }
        }
        n342 = Bundle By Name(cluster=w880, "VISA resource name"=w875) -> (w879:T11)
        n343 = call <vilib>:"Add State(s) to Queue__jki_lib_state_machine.vi"("State(s) in (\"\")"=w882) -> ("States Out"=w881:string)  [unwired: 14 in]
      }
      frame "Setup:RBDACOffset" {
        # "Your code here.\n(You can make a copy of, or modify, this frame)"
        n344 = Unbundle By Name(w963) -> ("VISA resource name"=w961:refnum<visa-resource-name>, "Connected?"=w957:bool, "Master Axis"=w956:i32, "Slave Axis"=w955:i32)
        n345 = case shown="True" w957 {
          tunnel: w961 -> [w966 w976]
          tunnel: w960 -> [w968 w978]
          tunnel: [w966 w975] -> w959
          tunnel: [w967 w973] -> w958
          tunnel: w956 -> [_ w972]
          tunnel: w955 -> [_ w971]
          frame False {
            n346 = call "Display Message to User3"("error in (no error)"=w968) -> ("error out"=w967:errorcluster)  [unwired: 9 in, 1 out]
          }
          frame True {
            n347 = Build Array(w972, w971) -> (w970:i32[])
            n348 = Sort 1D Array(array=w970) -> (sorted array=w969:i32[])
            n349 = for {
              tunnel: w978 -> [w989]
              tunnel: [w988] -> w974 mode=indexing
              tunnel: [w987] -> w977 mode=indexing
              tunnel: w976 -> [w986]
              tunnel: [w985] -> w975
              tunnel: w969 -> [w980] mode=indexing
              n350 = Decrement(x=w980) -> (x-1=w982:i32)
              n351 = Multiply(x=2, y=w982) -> (x*y=w983:i32)
              n352 = Add(x=1, y=w983) -> (x+y=w979:i32)
              n353 = call <instrlib>:"Get DAC Offset.vi"("error in (no error)"=w989, "Axis (1)"=w979, "VISA resource name"=w986) -> ("error out"=w988:errorcluster, "DAC Offset"=w987:dbl, "VISA resource name out"=w985:refnum<visa-resource-name>)  [unwired: 2 in]
            }
            "DAC Offsets" <- w977
            n354 = Merge Errors(w974) -> (w973:errorcluster)
          }
        }
        n355 = Bundle By Name(cluster=w963, "VISA resource name"=w959) -> (w962:T11)
        n356 = call <vilib>:"Add State(s) to Queue__jki_lib_state_machine.vi"("State(s) in (\"\")"=w965) -> ("States Out"=w964:string)  [unwired: 14 in]
      }
      frame "Setup:SetDACOffset" {
        # "Your code here.\n(You can make a copy of, or modify, this frame)"
        n357 = Unbundle By Name(w997) -> ("VISA resource name"=w995:refnum<visa-resource-name>, "Connected?"=w991:bool)
        n358 = case shown="True" w991 {
          tunnel: w995 -> [w1001 w1015]
          tunnel: w994 -> [w1003 w1013]
          tunnel: [w1001 w1011] -> w993
          tunnel: [w1002 w1012] -> w992
          tunnel: ["" "Setup:RBDACOffset" ("State(s) at Back (\"\")")] -> w990
          frame False {
            n359 = call "Display Message to User4"("error in (no error)"=w1003) -> ("error out"=w1002:errorcluster)  [unwired: 9 in, 1 out]
          }
          frame True {
            n360 = property on="AXIS" class="Ring (strict)"() -> ("Value"=w1009:i32)  [unwired: 2 in, 2 out]
            n361 = Decrement(x=w1009) -> (x-1=w1007:i32)
            n362 = Multiply(x=2, y=w1007) -> (x*y=w1006:i32)
            n363 = Add(x=1, y=w1006) -> (x+y=w1004:i32)
            n364 = call <instrlib>:"Set DAC Offset.vi"("error in (no error)"=w1013, "DAC Offset (0)"="DAC Offset (0)", "Axis (1)"=w1004, "VISA resource name"=w1015) -> ("error out"=w1012:errorcluster, "VISA resource name out"=w1011:refnum<visa-resource-name>)  [unwired: 2 in]
          }
        }
        n365 = Bundle By Name(cluster=w997, "VISA resource name"=w993) -> (w996:T11)
        n366 = call <vilib>:"Add State(s) to Queue__jki_lib_state_machine.vi"("State(s) in (\"\")"=w999, "State(s) at Back (\"\")"=w990) -> ("States Out"=w998:string)  [unwired: 13 in]
      }
      frame "Setup:RBGroup" {
        # "Template Separator\n(You can make a copy of, or modify, this frame)"
        n367 = Unbundle By Name(w1032) -> ("VISA resource name"=w1035:refnum<visa-resource-name>, "Group Cluster.Group Number (1)"=w1018:i32)
        n368 = call <instrlib>:"Get Group Velocity.vi"("error in (no error)"=w1030, "Group Number (1)"=w1018, "VISA resource name"=w1035) -> ("error out"=w1026:errorcluster, "Velocity (units/s)"=w1029:dbl, "VISA resource name out"=w1034:refnum<visa-resource-name>)  [unwired: 2 in]
        n369 = property on="Group Velocity (units/s)" class="DigNum (strict)"(error in=w1026, "Value"=w1029) -> (error out=w1025:errorcluster)  [unwired: 1 in, 1 out]
        n370 = call <instrlib>:"Get Group Acceleration.vi"("error in (no error)"=w1025, "Group Number (1)"=w1018, "VISA resource name"=w1034) -> ("error out"=w1024:errorcluster, "Acceleration (units/s²)"=w1028:dbl, "VISA resource name out"=w1033:refnum<visa-resource-name>)  [unwired: 2 in]
        n371 = property on="Group Acceleration\n (0 units/s²)" class="DigNum (strict)"(error in=w1024, "Value"=w1028) -> (error out=w1023:errorcluster)  [unwired: 1 in, 1 out]
        n372 = call <instrlib>:"Get Group Jerk.vi"("error in (no error)"=w1023, "Group Number (1)"=w1018, "VISA resource name"=w1033) -> ("error out"=w1022:errorcluster, "Jerk (units/s^3)"=w1027:dbl, "VISA resource name out"=w1020:refnum<visa-resource-name>)  [unwired: 2 in]
        n373 = property on="Group Vector Jerk\n (0 units/s^3)" class="DigNum (strict)"(error in=w1022, "Value"=w1027) -> (error out=w1017:errorcluster)  [unwired: 1 in, 1 out]
        n374 = call <instrlib>:"Get Group Decceleration.vi"("error in (no error)"=w1017, "Group Number (1)"=w1018, "VISA resource name"=w1020) -> ("error out"=w1016:errorcluster, "Decceleration (units/s²)"=w1021:dbl, "VISA resource name out"=w1019:refnum<visa-resource-name>)  [unwired: 2 in]
        n375 = property on="Group Decceleration \n(0 units/s²)" class="DigNum (strict)"("Value"=w1021) -> ()  [unwired: 2 in, 2 out]
        n376 = Bundle By Name(cluster=w1032, "VISA resource name"=w1019) -> (w1031:T11)
        n377 = call <vilib>:"Add State(s) to Queue__jki_lib_state_machine.vi"("State(s) in (\"\")"=w1037) -> ("States Out"=w1036:string)  [unwired: 14 in]
      }
      frame "Setup:KillGroups" {
        # "Template Separator\n(You can make a copy of, or modify, this frame)"
        n378 = Unbundle By Name(w1048) -> ("VISA resource name"=w1046:refnum<visa-resource-name>)
        n379 = call <instrlib>:"Get list of Groups Assigned.vi"("error in (no error)"=w1044, "VISA resource name"=w1046) -> ("error out"=w1042:errorcluster, "List of Groups"=w1045:string, "VISA resource name out"=w1041:refnum<visa-resource-name>)  [unwired: 3 in]
        n380 = call <instrlib>:"Error Query.vi"("VISA resource name"=w1041) -> ("error out"=w1039:errorcluster, "VISA resource name out"=w1040:refnum<visa-resource-name>)  [unwired: 3 in, 2 out]
        n381 = case shown="No Error" w1039 {
          tunnel: w1045 -> [w1059 _]
          tunnel: [w1054 w1066] -> w1043
          tunnel: w1042 -> [w1053 w1067]
          tunnel: [w1052 w1067] -> w1038
          tunnel: w1040 -> [w1051 w1066]
          frame No Error {
            n382 = call <vilib>:"Space Constant.vi"() -> ("String"=w1058:string)
            n383 = Spreadsheet String To Array(delimiter (Tab)=w1058, format string="", spreadsheet string=w1059, array type (2D Dbl)=string[] []) -> (array=w1056:string[])
            n384 = Decimal String To Number(string=w1056) -> (number=w1055:i32[])  [unwired: 2 in, 1 out]
            n385 = for {
              tunnel: w1055 -> [w1065] mode=indexing
              tunnel: w1051 -> [w1064]
              tunnel: [w1063] -> w1054
              shift-right: [w1061] -> w1052
              shift-left: w1053 -> [w1062]
              n386 = call <instrlib>:"Delete Group.vi"("error in (no error)"=w1062, "Group Number (1)"=w1065, "VISA resource name"=w1064) -> ("error out"=w1061:errorcluster, "VISA resource name out"=w1063:refnum<visa-resource-name>)  [unwired: 3 in]
            }
          }
          frame Error {
          }
        }
        n387 = Bundle By Name(cluster=w1048, "VISA resource name"=w1043) -> (w1047:T11)
        n388 = call <vilib>:"Add State(s) to Queue__jki_lib_state_machine.vi"("State(s) in (\"\")"=w1050) -> ("States Out"=w1049:string)  [unwired: 14 in]
      }
      frame "---------Connection---------" {
        # "Template Separator\n(You can make a copy of, or modify, this frame)"
        n389 = call <vilib>:"Add State(s) to Queue__jki_lib_state_machine.vi"("State(s) in (\"\")"=w1071) -> ("States Out"=w1070:string)  [unwired: 14 in]
      }
      frame "Connection:Errorcheck" {
        # "Template Separator\n(You can make a copy of, or modify, this frame)"
        n390 = Unbundle By Name(w1076) -> ("VISA resource name"=w1078:refnum<visa-resource-name>)
        n391 = call <instrlib>:"Error Query.vi"("error in (no error)"=w1077, "VISA resource name"=w1078) -> ("error out"=w1072:errorcluster, "VISA resource name out"=w1074:refnum<visa-resource-name>)  [unwired: 2 in, 2 out]
        n392 = case shown="Error" w1072 {
          tunnel: w1073 -> [_ w1080]
          frame No Error {
          }
          frame Error {
            "Remaining States" <- w1080
          }
        }
        n393 = Bundle By Name(cluster=w1076, "VISA resource name"=w1074) -> (w1075:T11)
        n394 = call <vilib>:"Add State(s) to Queue__jki_lib_state_machine.vi"("State(s) in (\"\")"=w1073) -> ("States Out"=w1079:string)  [unwired: 14 in]
      }
      frame "Connection:Init" {
        # "Your code here.\n(You can make a copy of, or modify, this frame)"
        n395 = Unbundle By Name(w1090) -> ()  [unwired: 1 out]
        n396 = call <instrlib>:"Initialize.vi"("VISA resource name"="VISA resource name", "ID Query (True)"=FALSE, "Reset (False)"=FALSE, "error in (no error)"=w1093, "Serial Link (RS232)"="Serial Link (RS232)") -> ("VISA resource name out"=w1081:refnum<visa-resource-name>, "error out"=w1082:errorcluster)  [unwired: 4 in]
        n397 = case shown="Error" w1082 {
          selector: w1082 -> [w1098 w1101]
          tunnel: [w1098 w1100] -> w1091
          tunnel: w1081 -> [w1097 w1105]
          tunnel: [w1097 w1105] -> w1088
          tunnel: [TRUE ("Reset (False)") w1104] -> w1085
          tunnel: ["Setup:RBSetup\nSetup:RBFBFilter\nSetup:RBDACOffset\nSetup:InitButtons\nSetup:MotorONOFF>>ON\nSetup:RBMotorPower\nSetup:KillGroups" ("State(s) at Back (\"\")") ""] -> w1086
          frame No Error {
          }
          frame Error {
            w1104 = FALSE ("Reset (False)")
            n398 = property on="Connect" class="Bool (strict)"("Value"=w1104) -> (error out=w1102:errorcluster)  [unwired: 2 in, 1 out]
            n399 = Merge Errors(w1101, w1102) -> (w1100:errorcluster)
          }
        }
        "Connected?" <- w1085
        n400 = Bundle By Name(cluster=w1090, "VISA resource name"=w1088, "Connected?"=w1085) -> (w1089:T11)
        n401 = call <vilib>:"Add State(s) to Queue__jki_lib_state_machine.vi"("State(s) in (\"\")"=w1095, "State(s) at Back (\"\")"=w1086) -> ("States Out"=w1094:string)  [unwired: 13 in]
      }
      frame "Connection:Close" {
        w1108 = FALSE ("Connected?")
        # "Your code here.\n(You can make a copy of, or modify, this frame)"
        n402 = Unbundle By Name(w1111) -> ("VISA resource name"=w1107:refnum<visa-resource-name>)
        n403 = call <instrlib>:"Close.vi"("error in (no error)"=w1106, "VISA resource name"=w1107) -> ("error out"=w1109:errorcluster)  [unwired: 9 in]
        n404 = property on="Connected?" class="Bool (strict)"("Value"=w1108) -> ()  [unwired: 2 in, 2 out]
        n405 = Bundle By Name(cluster=w1111, "Connected?"=w1108) -> (w1110:T11)
        n406 = call <vilib>:"Add State(s) to Queue__jki_lib_state_machine.vi"("State(s) in (\"\")"=w1113) -> ("States Out"=w1112:string)  [unwired: 14 in]
      }
      frame "--------Motion---------" {
        # "Template Separator\n(You can make a copy of, or modify, this frame)"
        n407 = call <vilib>:"Add State(s) to Queue__jki_lib_state_machine.vi"("State(s) in (\"\")"=w1117) -> ("States Out"=w1116:string)  [unwired: 14 in]
      }
      frame "Motion:MasterMove" {
        # "Template Separator\n(You can make a copy of, or modify, this frame)"
        n408 = Unbundle By Name(w1128) -> ("VISA resource name"=w1126:refnum<visa-resource-name>, "Master Axis"=w1127:i32, "Connected?"=w1121:bool, "Group Cluster.Grouped?"=w1120:bool, "Group Cluster.Group Number (1)"=w1119:i32, "In Motion?"=w1118:bool)
        n409 = case shown="True" w1121 {
          tunnel: w1126 -> [w1134 w1145]
          tunnel: w1127 -> [_ w1144]
          tunnel: [w1134 w1137] -> w1125
          tunnel: w1123 -> [w1132 w1142]
          tunnel: [w1132 w1135] -> w1122
          tunnel: [FALSE w1141] -> w1124
          tunnel: w1120 -> [_ _]
          tunnel: w1119 -> [_ _]
          tunnel: w1118 -> [_ w1141]
          frame False {
          }
          frame True {
            n410 = property on="MOVE MASTER" class="Bool (strict)"() -> ("Value"=w1143:bool)  [unwired: 2 in, 2 out]
            n411 = Not(x=w1141) -> (.not. x?=w1139:bool)
            n412 = Or(x=w1139, y=w1143) -> (x .or. y?=w1140:bool)
            n413 = case shown="False" w1140 {
              tunnel: w1145 -> [w1157 w1159]
              tunnel: w1144 -> [w1156 _]
              tunnel: [w1155 w1159] -> w1138
              tunnel: w1142 -> [w1154 w1158]
              tunnel: [w1153 w1158] -> w1136
              frame False {
                n414 = call <instrlib>:"Stop Motion.vi"("error in (no error)"=w1154, "Stop all axes (F)"=TRUE, "Axis (1)"=w1156, "VISA resource name"=w1157) -> ("error out"=w1153:errorcluster, "VISA resource name out"=w1155:refnum<visa-resource-name>)  [unwired: 2 in]
              }
              frame True {
              }
            }
            n415 = disable-structure shown="Enabled" {
              disable-tunnel: w1138 -> [w1149 w1151]
              disable-tunnel: [w1148 w1151] -> w1137
              disable-tunnel: w1136 -> [w1147 w1150]
              disable-tunnel: [w1146 w1150] -> w1135
              frame Disabled {
                n416 = call <instrlib>:"Error Query.vi"("error in (no error)"=w1147, "VISA resource name"=w1149) -> ("error out"=w1146:errorcluster, "VISA resource name out"=w1148:refnum<visa-resource-name>)  [unwired: 2 in, 2 out]
              }
              frame Enabled {
              }
            }
          }
        }
        "In Motion?" <- w1124
        n417 = Bundle By Name(cluster=w1128, "VISA resource name"=w1125) -> (w1129:T11)
        n418 = call <vilib>:"Add State(s) to Queue__jki_lib_state_machine.vi"("State(s) in (\"\")"=w1131) -> ("States Out"=w1130:string)  [unwired: 14 in]
      }
      frame "Motion:StepperMaster" {
        # "Template Separator\n(You can make a copy of, or modify, this frame)"
        n419 = Unbundle By Name(w1185) -> ("Master Axis"=w1175:i32, "Slave Axis"=w1183:i32, "VISA resource name"=w1174:refnum<visa-resource-name>, "Stepper Cluster.Moving"=w1168:bool, "Stepper Cluster.millisecond timer value"=w1178:u32, "Stepper Cluster.act. Step"=w1170:u32, "Stepper Cluster.Stepped Motion"=w1166:bool, "actual Position"=w1162:dbl, "Last Position"=w1160:dbl)
        n420 = Less?(x=w1170, y="Number of Steps") -> (x < y?=w1165:bool)
        n421 = And(x=w1166, y=w1165) -> (x .and. y?=w1164:bool)
        n422 = case shown="True" w1164 {
          selector: w1164 -> [w1191 w1202]
          tunnel: w1168 -> [_ w1209]
          tunnel: [0 ("f") w1207] -> w1181
          tunnel: [u32 0 ("millisecond timer value") w1206] -> w1180
          tunnel: w1178 -> [_ w1205]
          tunnel: w1175 -> [w1197 _]
          tunnel: w1174 -> [w1195 w1204]
          tunnel: [w1194 w1204] -> w1173
          tunnel: w1172 -> [w1193 w1203]
          tunnel: [w1188 w1203] -> w1171
          tunnel: [w1191 w1202] -> w1163
          tunnel: w1162 -> [_ w1200]
          tunnel: w1160 -> [_ w1199]
          frame False {
            n423 = call <instrlib>:"Stop Motion.vi"("error in (no error)"=w1193, "Stop all axes (F)"=TRUE, "Axis (1)"=w1197, "VISA resource name"=w1195) -> ("error out"=w1189:errorcluster, "VISA resource name out"=w1194:refnum<visa-resource-name>)  [unwired: 2 in]
            n424 = property on="Go steps" class="Bool (strict)"(error in=w1189, "Value"=FALSE ("Go steps")) -> (error out=w1188:errorcluster)  [unwired: 1 in, 1 out]
          }
          frame True {
            n425 = call "StepperDecision.vi"("Last Pos"=w1199, "Steplength(ms)"="Steplength(ms/mm)", "Waittime"="Waittime", "StepMode"="StepMode", "act Pos"=w1200, "millisecond timer value"=w1205, "Moving"=w1209) -> ("f"=w1207:i32, "millisecond timer value 2"=w1206:u32)  [unwired: 2 in]
          }
        }
        n426 = case shown="2" w1181 {
          tunnel: w1173 -> [w1216 w1227 w1255]
          tunnel: w1183 -> [_ w1225 w1254]
          tunnel: [w1216 w1226 w1253] -> w1182
          tunnel: w1180 -> [_ w1218 w1252]
          tunnel: w1178 -> [w1212 _ _]
          tunnel: [w1212 w1218 w1252] -> w1179
          tunnel: w1171 -> [w1215 w1224 w1251]
          tunnel: [w1215 w1221 w1247] -> w1177
          tunnel: w1170 -> [w1214 w1228 w1250]
          tunnel: [w1214 w1228 w1249] -> w1169
          tunnel: w1168 -> [w1213 _ _]
          tunnel: [w1213 FALSE ("Moving") TRUE ("Moving")] -> w1167
          tunnel: w1162 -> [_ w1217 w1246]
          tunnel: [w1211 w1217 w1246] -> w1161
          tunnel: w1160 -> [w1211 _ _]
          frame 0, Default {
          }
          frame 1 {
            n427 = flat-sequence {
              tunnel: w1227 -> [w1233]
              tunnel: [w1232] -> w1226
              tunnel: w1225 -> [w1231]
              tunnel: w1224 -> [w1230]
              tunnel: [w1229] -> w1222
              tunnel: [w1235] -> w1223
              tunnel: w1222 -> [w1235]
              tunnel: w1223 -> [w1238]
              tunnel: [w1237] -> w1219
              tunnel: [w1245] -> w1221
              tunnel: w1219 -> [w1245]
              frame #0 {
                n428 = call <instrlib>:"Set Master-Slave Reduction Ratio.vi"("error in (no error)"=w1230, "Reduction Ratio (0)"=1.0, "Axis (1)"=w1231, "VISA resource name"=w1233) -> ("error out"=w1229:errorcluster, "VISA resource name out"=w1232:refnum<visa-resource-name>)  [unwired: 2 in]
              }
              frame #1 {
                n429 = Wait (ms)(milliseconds to wait="Wait befor picture(ms)") -> ()  [unwired: 1 out]
              }
              frame #2 {
                n430 = case shown="True" "Make Pictures" {
                  selector: "Make Pictures" -> [_ w1243]
                  tunnel: w1238 -> [w1240 w1242]
                  tunnel: [w1240 w1241] -> w1237
                  frame False {
                  }
                  frame True {
                    n431 = property on="Save sinlge\nPicture" class="Bool (strict)"(error in=w1242, "Value"=w1243) -> (error out=w1241:errorcluster)  [unwired: 1 in, 1 out]
                  }
                }
              }
              frame #3 {
                n432 = Wait (ms)(milliseconds to wait="Wait after picture(ms) 2") -> ()  [unwired: 1 out]
              }
            }
          }
          frame 2 {
            n433 = Increment(x=w1250) -> (x+1=w1249:u32)
            n434 = call <instrlib>:"Set Master-Slave Reduction Ratio.vi"("error in (no error)"=w1251, "Reduction Ratio (0)"=0.0, "Axis (1)"=w1254, "VISA resource name"=w1255) -> ("error out"=w1247:errorcluster, "VISA resource name out"=w1253:refnum<visa-resource-name>)  [unwired: 2 in]
          }
        }
        "act. Step" <- w1169
        n435 = Bundle By Name(cluster=w1185, "VISA resource name"=w1182, "Stepper Cluster.millisecond timer value"=w1179, "Stepper Cluster.act. Step"=w1169, "Stepper Cluster.Moving"=w1167, "Stepper Cluster.Stepped Motion"=w1163, "Last Position"=w1161) -> (w1184:T11)
        n436 = call <vilib>:"Add State(s) to Queue__jki_lib_state_machine.vi"("State(s) in (\"\")"=w1187) -> ("States Out"=w1186:string)  [unwired: 14 in]
      }
      frame "Motion:StepperMaster2" {
        # "Template Separator\n(You can make a copy of, or modify, this frame)"
        n437 = Unbundle By Name(w1282) -> ("Master Axis"=w1260:i32, "Slave Axis"=w1280:i32, "VISA resource name"=w1272:refnum<visa-resource-name>, "Stepper Cluster 2.Moving"=w1266:bool, "Stepper Cluster 2.millisecond timer value"=w1275:u32, "Stepper Cluster 2.act. Step"=w1268:u32, "Stepper Cluster 2.Stepped Motion"=w1264:bool, "actual Position"=w1259:dbl, "Last Position"=w1258:dbl)
        n438 = Less?(x=w1268, y="Number of Steps 2") -> (x < y?=w1263:bool)
        n439 = And(x=w1264, y=w1263) -> (x .and. y?=w1262:bool)
        n440 = case shown="True" w1262 {
          selector: w1262 -> [w1288 w1299]
          tunnel: w1266 -> [_ w1306]
          tunnel: [0 ("f") w1304] -> w1278
          tunnel: [u32 0 ("millisecond timer value") w1303] -> w1277
          tunnel: w1275 -> [_ w1302]
          tunnel: w1260 -> [w1294 _]
          tunnel: w1272 -> [w1292 w1301]
          tunnel: [w1291 w1301] -> w1271
          tunnel: w1270 -> [w1290 w1300]
          tunnel: [w1285 w1300] -> w1269
          tunnel: [w1288 w1299] -> w1261
          tunnel: w1259 -> [_ w1298]
          tunnel: w1258 -> [_ w1297]
          frame False {
            n441 = call <instrlib>:"Stop Motion.vi"("error in (no error)"=w1290, "Stop all axes (F)"=TRUE, "Axis (1)"=w1294, "VISA resource name"=w1292) -> ("error out"=w1286:errorcluster, "VISA resource name out"=w1291:refnum<visa-resource-name>)  [unwired: 2 in]
            n442 = property on="Go steps 2" class="Bool (strict)"(error in=w1286, "Value"=FALSE ("Go steps")) -> (error out=w1285:errorcluster)  [unwired: 1 in, 1 out]
          }
          frame True {
            n443 = property on="StepMode" class="Enum (strict)"() -> ("Value"=w1296:enum16{"Use Timing", "Use Encoder"})  [unwired: 2 in, 2 out]
            n444 = call "StepperDecision.vi"("Last Pos"=w1297, "Steplength(ms)"="Steplength(ms) 2", "Waittime"="Waittime 2", "StepMode"=w1296, "act Pos"=w1298, "millisecond timer value"=w1302, "Moving"=w1306) -> ("f"=w1304:i32, "millisecond timer value 2"=w1303:u32)  [unwired: 2 in]
          }
        }
        n445 = case shown="0, Default" w1278 {
          tunnel: w1271 -> [w1313 w1324 w1357]
          tunnel: w1280 -> [_ w1322 w1355]
          tunnel: [w1313 w1323 w1351] -> w1279
          tunnel: w1277 -> [_ w1326 _]
          tunnel: w1275 -> [w1312 _ w1348]
          tunnel: [w1312 w1326 w1348] -> w1276
          tunnel: w1269 -> [w1311 w1321 w1353]
          tunnel: [w1311 w1318 w1352] -> w1274
          tunnel: w1268 -> [w1310 w1325 w1360]
          tunnel: [w1310 w1325 w1359] -> w1267
          tunnel: w1266 -> [w1309 _ _]
          tunnel: [w1309 FALSE ("Moving") TRUE ("Moving")] -> w1265
          tunnel: w1260 -> [_ w1315 w1356]
          tunnel: w1259 -> [_ w1314 w1347]
          tunnel: w1258 -> [w1308 _ _]
          tunnel: [w1308 w1314 w1347] -> w1257
          frame 0, Default {
          }
          frame 1 {
            n446 = flat-sequence {
              tunnel: w1324 -> [w1329]
              tunnel: [w1335] -> w1323
              tunnel: w1322 -> [w1331]
              tunnel: w1321 -> [w1332]
              tunnel: [w1334] -> w1319
              tunnel: w1315 -> [w1330]
              tunnel: [w1336] -> w1320
              tunnel: w1319 -> [w1336]
              tunnel: w1320 -> [w1339]
              tunnel: [w1338] -> w1316
              tunnel: [w1346] -> w1318
              tunnel: w1316 -> [w1346]
              frame #0 {
                n447 = call "comp_stop2.vi"("VISA resource name"=w1329, "Master Axis"=w1330, "Slave Axis"=w1331, "Reduction Ratio (0)"=1.0, "error in (no error)"=w1332, "Velocity (units/s)"="Stiff Velo", "Acceleration (0 units/s²)"="Stiff Acc") -> ("VISA resource name out"=w1335:refnum<visa-resource-name>, "error out"=w1334:errorcluster)  [unwired: 7 in]
              }
              frame #1 {
                n448 = Wait (ms)(milliseconds to wait="Wait befor\n picture(ms) 2") -> ()  [unwired: 1 out]
              }
              frame #2 {
                n449 = case shown="True" "Make Pictures 2" {
                  selector: "Make Pictures 2" -> [_ w1344]
                  tunnel: w1339 -> [w1341 w1343]
                  tunnel: [w1341 w1342] -> w1338
                  frame False {
                  }
                  frame True {
                    n450 = property on="Save sinlge\nPicture" class="Bool (strict)"(error in=w1343, "Value"=w1344) -> (error out=w1342:errorcluster)  [unwired: 1 in, 1 out]
                  }
                }
              }
              frame #3 {
                n451 = Wait (ms)(milliseconds to wait="Wait after\n picture(ms) 2") -> ()  [unwired: 1 out]
              }
            }
          }
          frame 2 {
            n452 = call "comp_stop2.vi"("VISA resource name"=w1357, "Master Axis"=w1356, "Slave Axis"=w1355, "Reduction Ratio (0)"=0.0, "error in (no error)"=w1353, "Velocity (units/s)"="Step Velo", "Acceleration (0 units/s²)"="Step Acc") -> ("VISA resource name out"=w1351:refnum<visa-resource-name>, "error out"=w1352:errorcluster)  [unwired: 7 in]
            n453 = Increment(x=w1360) -> (x+1=w1359:u32)
          }
        }
        "act. Step 2" <- w1267
        n454 = Bundle By Name(cluster=w1282, "VISA resource name"=w1279, "Stepper Cluster 2.millisecond timer value"=w1276, "Stepper Cluster 2.act. Step"=w1267, "Stepper Cluster 2.Moving"=w1265, "Stepper Cluster 2.Stepped Motion"=w1261, "Last Position"=w1257) -> (w1281:T11)
        n455 = call <vilib>:"Add State(s) to Queue__jki_lib_state_machine.vi"("State(s) in (\"\")"=w1284) -> ("States Out"=w1283:string)  [unwired: 14 in]
      }
      frame "Motion:StepperMaster3" {
        # "Template Separator\n(You can make a copy of, or modify, this frame)"
        n456 = Unbundle By Name(w1389) -> ("Master Axis"=w1367:i32, "Slave Axis"=w1387:i32, "VISA resource name"=w1379:refnum<visa-resource-name>, "Stepper Cluster 3.Moving"=w1373:bool, "Stepper Cluster 3.millisecond timer value"=w1382:u32, "Stepper Cluster 3.act. Step"=w1375:u32, "Stepper Cluster 3.Stepped Motion"=w1371:bool, "Group Cluster.Group Number (1)"=w1366:i32, "Group Cluster"=w1365:T10, "actual Position"=w1364:dbl, "Last Position"=w1363:dbl)
        n457 = Less?(x=w1375, y="Number of Steps 3") -> (x < y?=w1370:bool)
        n458 = And(x=w1371, y=w1370) -> (x .and. y?=w1369:bool)
        n459 = case shown="True" w1369 {
          selector: w1369 -> [w1396 w1405]
          tunnel: w1373 -> [_ w1412]
          tunnel: [0 ("f") w1410] -> w1385
          tunnel: [u32 0 ("millisecond timer value") w1409] -> w1384
          tunnel: w1382 -> [_ w1408]
          tunnel: w1379 -> [w1400 w1407]
          tunnel: [w1399 w1407] -> w1378
          tunnel: w1377 -> [w1398 w1406]
          tunnel: [w1393 w1406] -> w1376
          tunnel: [w1396 w1405] -> w1368
          tunnel: w1366 -> [w1392 _]
          tunnel: w1364 -> [_ w1404]
          tunnel: w1363 -> [_ w1403]
          frame False {
            n460 = call <instrlib>:"Stop Group Motion.vi"("error in (no error)"=w1398, "Group Number (1)"=w1392, "VISA resource name"=w1400) -> ("error out"=w1394:errorcluster, "VISA resource name out"=w1399:refnum<visa-resource-name>)  [unwired: 3 in]
            n461 = property on="Go steps 3" class="Bool (strict)"(error in=w1394, "Value"=FALSE ("Go steps")) -> (error out=w1393:errorcluster)  [unwired: 1 in, 1 out]
          }
          frame True {
            n462 = property on="StepMode" class="Enum (strict)"() -> ("Value"=w1402:enum16{"Use Timing", "Use Encoder"})  [unwired: 2 in, 2 out]
            n463 = call "StepperDecision.vi"("Last Pos"=w1403, "Steplength(ms)"="Steplength(ms) 3", "Waittime"="Waittime 3", "StepMode"=w1402, "act Pos"=w1404, "millisecond timer value"=w1408, "Moving"=w1412) -> ("f"=w1410:i32, "millisecond timer value 2"=w1409:u32)  [unwired: 2 in]
          }
        }
        n464 = case shown="1" w1385 {
          tunnel: w1378 -> [w1420 w1433 w1470]
          tunnel: w1387 -> [_ w1431 w1460]
          tunnel: [w1420 w1432 w1461] -> w1386
          tunnel: w1384 -> [_ w1435 w1458]
          tunnel: w1382 -> [w1419 _ _]
          tunnel: [w1419 w1435 w1458] -> w1383
          tunnel: w1376 -> [w1418 w1430 w1468]
          tunnel: [w1418 w1427 w1459] -> w1381
          tunnel: w1375 -> [w1417 w1434 w1473]
          tunnel: [w1417 w1434 w1472] -> w1374
          tunnel: w1373 -> [w1416 _ _]
          tunnel: [w1416 FALSE ("Moving") TRUE ("Moving")] -> w1372
          tunnel: w1367 -> [_ w1424 w1465]
          tunnel: w1365 -> [_ w1423 w1463]
          tunnel: w1364 -> [_ w1422 w1457]
          tunnel: w1363 -> [w1415 _ _]
          tunnel: [w1415 w1422 w1457] -> w1362
          tunnel: ["" "Setup:GroupSpeed" ""] -> w1361
          frame 0, Default {
          }
          frame 1 {
            n465 = flat-sequence {
              tunnel: w1433 -> [w1444]
              tunnel: [w1443] -> w1432
              tunnel: w1431 -> [w1441]
              tunnel: w1430 -> [w1438]
              tunnel: [w1442] -> w1428
              tunnel: w1424 -> [w1440]
              tunnel: w1423 -> [w1439]
              tunnel: [w1445] -> w1429
              tunnel: w1428 -> [w1445]
              tunnel: w1429 -> [w1448]
              tunnel: [w1447] -> w1425
              tunnel: [w1455] -> w1427
              tunnel: w1425 -> [w1455]
              frame #0 {
                n466 = control-ref of="E Stop"() -> (w1436:refnum<vi>)
                n467 = call "Comp_Group_Motion.vi"("stop 2"=w1436, "Slave Axis"=w1441, "Master Axis"=w1440, "error in (no error)"=w1438, "Motionphase"="Motionphase", "Group Cluster"=w1439, "VISA resource name in"=w1444) -> ("error out"=w1442:errorcluster, "VISA resource name out"=w1443:refnum<visa-resource-name>)  [unwired: 3 in]
              }
              frame #1 {
                n468 = Wait (ms)(milliseconds to wait="Wait befor\n picture(ms) 3") -> ()  [unwired: 1 out]
              }
              frame #2 {
                n469 = case shown="True" "Make Pictures 3" {
                  selector: "Make Pictures 3" -> [_ w1453]
                  tunnel: w1448 -> [w1450 w1452]
                  tunnel: [w1450 w1451] -> w1447
                  frame False {
                  }
                  frame True {
                    n470 = property on="Save sinlge\nPicture" class="Bool (strict)"(error in=w1452, "Value"=w1453) -> (error out=w1451:errorcluster)  [unwired: 1 in, 1 out]
                  }
                }
              }
              frame #3 {
                n471 = Wait (ms)(milliseconds to wait="Wait after\n picture(ms) 3") -> ()  [unwired: 1 out]
              }
            }
          }
          frame 2 {
            n472 = Unbundle By Name(w1463) -> ("Group Number (1)"=w1469:i32)
            n473 = call <instrlib>:"Stop Group Motion.vi"("error in (no error)"=w1468, "Group Number (1)"=w1469, "VISA resource name"=w1470) -> ("error out"=w1467:errorcluster, "VISA resource name out"=w1462:refnum<visa-resource-name>)  [unwired: 3 in]
            n474 = property on="1st Holdmove" class="DigNum (strict)"() -> ("Value"=w1464:dbl)  [unwired: 2 in, 2 out]
            n475 = Increment(x=w1473) -> (x+1=w1472:u32)
            n476 = call "ESP301GroupMove.vi"("VISA resource name"=w1462, "Slave Axis"=w1460, "Group Cluster"=w1463, "MaxMotion"=w1464, "Master Axis"=w1465, "error in"=w1467, "Reduction"=0.0) -> ("VISA resource name out"=w1461:refnum<visa-resource-name>, "error out"=w1459:errorcluster)  [unwired: 7 in]
          }
        }
        "act. Step 3" <- w1374
        n477 = Bundle By Name(cluster=w1389, "VISA resource name"=w1386, "Stepper Cluster 3.millisecond timer value"=w1383, "Stepper Cluster 3.act. Step"=w1374, "Stepper Cluster 3.Moving"=w1372, "Stepper Cluster 3.Stepped Motion"=w1368, "Last Position"=w1362) -> (w1388:T11)
        n478 = call <vilib>:"Add State(s) to Queue__jki_lib_state_machine.vi"("State(s) in (\"\")"=w1391, "State(s) at Back (\"\")"=w1361) -> ("States Out"=w1390:string)  [unwired: 13 in]
      }
    }
    n479 = Unbundle By Name(w5) -> ("Master Axis"=→"Master Axis":i32, "Slave Axis"=→"Slave Axis":i32)
  }
  n480 = disable-structure shown="Disabled" {
    frame Disabled {
      n481 = call <instrlib>:"Set Trajectory Mode.vi"() -> ()  [unwired: 7 in, 2 out]
      n482 = control-ref of="E Stop"() -> ()  [unwired: 1 out]
      n483 = call <instrlib>:"Move Relative.vi"() -> ()  [unwired: 6 in, 2 out]
      n484 = call "ESP301GroupMove.vi"() -> ()  [unwired: 14 in, 2 out]
      n485 = property on="Encoder\nAxis" class="DigNum (strict)" props=["Value"]() -> ()  [unwired: 2 in, 3 out]
    }
    frame Enabled {
    }
  }
